vi "STED Control V8.vi"() -> ()   [LabVIEW 2014]
uses:
  Type Defs/Image Acquisition Parameters.ctl
  Laser Controls.ctl
  Detectors.ctl
  Type Defs/P541.ctl
  Type Defs/M227.ctl
  Type Defs/P612.ctl
  Type Defs/M686.ctl
  Type Defs/P841.ctl
  Type Defs/ASI.ctl
  Type Defs/N664_V2.ctl
  Type Defs/STED Graph Controls.ctl
  Type Defs/Display Controls.ctl
  FPGA-7842R-Reference.ctl
  Manual Controls V2.ctl
  Scan Parameters.ctl
  <vilib>/Utility/miscctls.llb/LVPositionTypeDef.ctl
  Controls/StageStates.ctl
  <vilib>/Utility/miscctls.llb/LVRectTypeDef.ctl
  <vilib>/event_ctls.llb/lveventtype.ctl
panel:
  out "Channel 6":sgl[][](graph)
  out "Channel 5":sgl[][](graph)
  out "Channel 4":sgl[][](graph)
  out "Channel 3":sgl[][](graph)
  out "Channel 2":sgl[][](graph)
  out "Channel 1":sgl[][](graph)
  in  "Display Controls":T1
  in  "Graph Tools":T2
  in  "Shutters":T3
  in  "Upper Objective Z - N664":T4={"Up N664"=FALSE, "Down N664"=FALSE, "Step Size (um)"=0.001, "Position (mm)"=0.0} {"Step Size (um)" min=0.001}
  in  "Load Positions":bool
  in  "Cavity Translation Z - ASI":T5={"Up ASI"=FALSE, "Down ASI"=FALSE, "Step Size (um)"=0.001, "Z (um)"=0.001, "F (um)"=0.001, "Velocity"=0.001} caption="ASI" {"Velocity" min=0.001; "F (um)" min=0.001; "Z (um)" min=-1500.0 max=1500.0; "Step Size (um)" min=0.001}
  in  "Phase Comp Mirror - P841":T6={"Position (µm)"=0.0, "Step Size (µm)"=1.0, "Up P841"=FALSE, "Down P841"=FALSE}
  in  "Sample Stage XY - M686":T7 {"Y" format="%#_4g"; "X" format="%#_4g"}
  in  "Joystick Velocity":string(combo)
  in  "Radio Buttons":enum32{"Radio Selection 1", "Radio Selection 2"}(radio)
  in  "Bottom Objective XY - P612":T8 {"Y" format="%#_4g"; "X" format="%#_4g"}
  in  "Abort AllStage":bool
  in  "Stages":T9={"M227"=TRUE, "N664"=TRUE, "P612"=TRUE, "M686"=TRUE, "P841"=TRUE, "ASI"=TRUE}
  in  "Sample Z Coarse - M227":T10
  in  "Tab Control":T11(tab)
  in  "SLM":bool
  in  "DM":bool
  in  "Timing":bool
  in  "Sample Z - P541":T12={"Step Up"=FALSE, "Step Down"=FALSE, "Z Position"=0.0, "Step Size (um)"=1.0}
  in  "Detectors":T13
  in  "Laser Controls":T14 {"STED Power (V)" scale=0.0..2.0}
  in  "Save File Path":path=path "C:/isoSTED_Data/Temp/Test_0000.dbl"
  in  "Capture":bool
  in  "Image Acquisition Parameters":T15={"Scan Type"=enum."Beam Scanning", "Scan Mode"=enum."XY", "Fast Axis Frequency (Hz)"=15780.0, "Image Format"=256, "Line Accumulations"=100, "Frames Per Capture"=1, "Frames Accumulations"=1, "Image Dimension (um)"=[15.0, 15.0], "Number of Z Steps"=1, "Z Steps Size (um)"=1.0, "Pixel Size (nm)"=[58.59375, 58.59375]} {"Z Steps Size (um)" min=0.0; "Number of Z Steps" min=1; "Frames Accumulations" min=1; "Frames Per Capture" min=1; "Line Accumulations" min=1; "Image Format" items=["64 x 64"=64, "128 x 128"=128, "256 x 256"=256, "512 x 512"=512, "1024 x 1024"=1024, "2048 x 2048"=2048]}
  in  "Live":bool
  in  "Exit":bool
  # "Sample Stage XY - M686 (0~25 mm)"
  # "XY"
  # "Z"
  # "Length"
  # "Height"
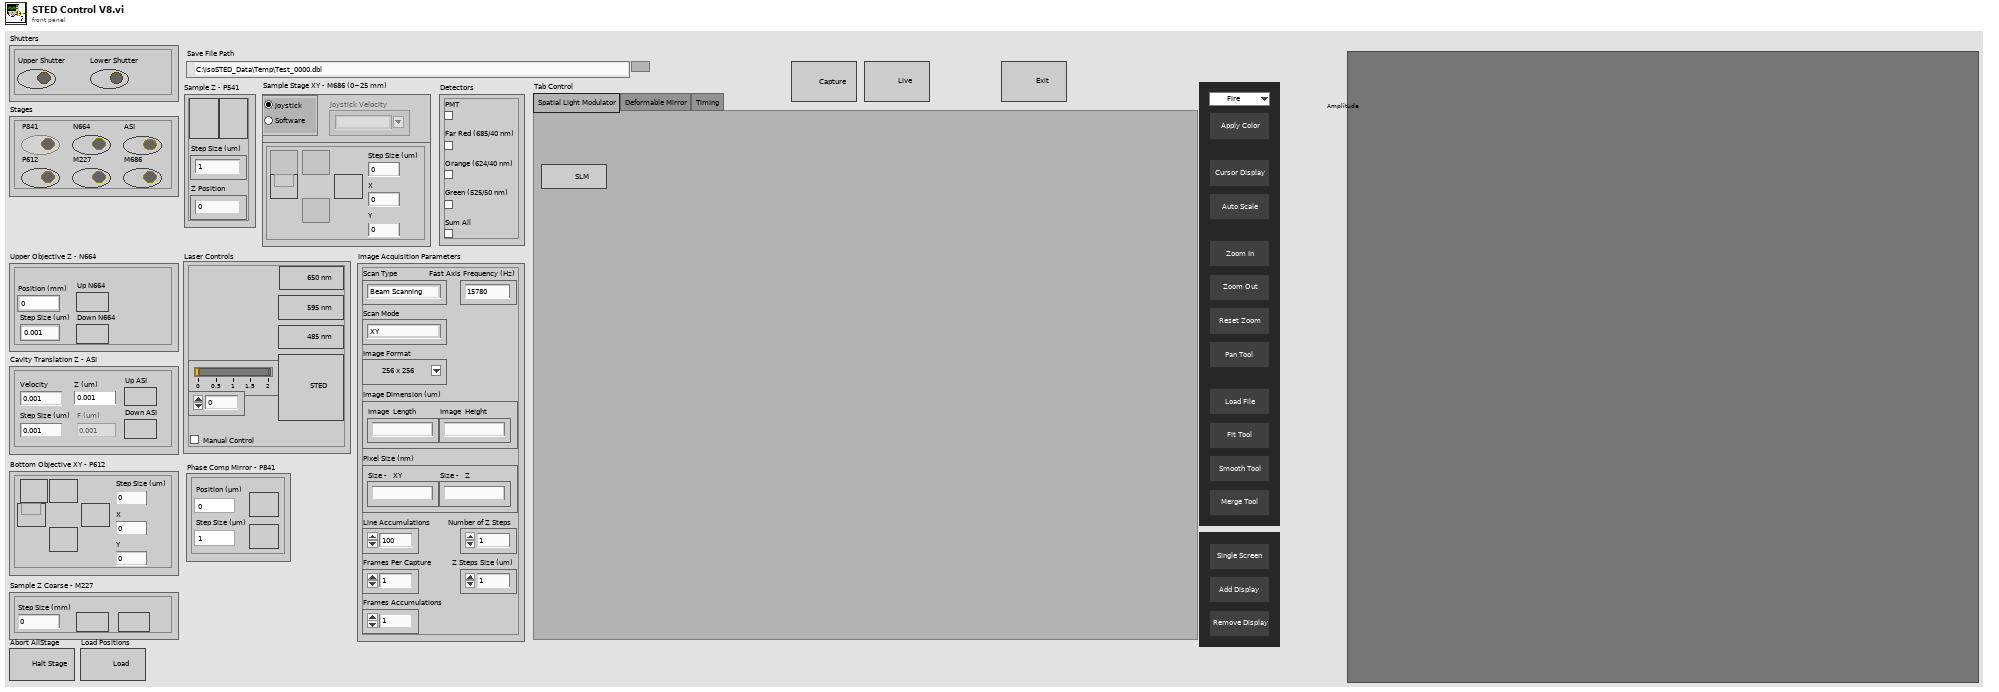
[diagram p1: front panel]
types:
  T1 = typedef "Display Controls.ctl" = cluster{"Remove Display":bool, "Add Display":bool, "Single Screen":bool}
  T2 = typedef "STED Graph Controls.ctl" = cluster{"Zoom Out":bool, "Zoom In":bool, "Reset Zoom":bool, "Pan Tool":bool, "Show Cursor":bool, "Load File":bool, "Fit Tool":bool, "Smooth Tool":bool, "Merge Tool":bool, "Auto Scale":bool, "Apply Color":bool, "Color Map":enum16{"Fire", "Gray", "Red", "Green", "Blue", "Cyan", "Magenta", "Yellow", "Red-White", "Green-White", "Blue-White", "Glow"}}
  T3 = cluster{"Upper Shutter":bool, "Lower Shutter":bool}
  T4 = typedef "N664_V2.ctl" = cluster{"Up N664":bool, "Down N664":bool, "Step Size (um)":dbl, "Position (mm)":dbl}
  T5 = typedef "ASI.ctl" = cluster{"Up ASI":bool, "Down ASI":bool, "Step Size (um)":dbl, "Z (um)":dbl, "F (um)":dbl, "Velocity":dbl}
  T6 = typedef "P841.ctl" = cluster{"Position (µm)":dbl, "Step Size (µm)":dbl, "Up P841":bool, "Down P841":bool}
  T7 = typedef "M686.ctl" = cluster{"Home Button":bool, "Up Button":bool, "Left Button":bool, "Down Button":bool, "Right Button":bool, "Step Size (um)":dbl, "X":dbl, "Y":dbl}
  T8 = typedef "P612.ctl" = cluster{"Home Button":bool, "Up Button":bool, "Left Button":bool, "Down Button":bool, "Right Button":bool, "Step Size (um)":dbl, "X":dbl, "Y":dbl}
  T9 = cluster{"M227":bool, "N664":bool, "P612":bool, "M686":bool, "P841":bool, "ASI":bool}
  T10 = typedef "M227.ctl" = cluster{"Up M227":bool, "Down M227":bool, "Step Size (mm)":dbl}
  T11 = enum32{"Spatial Light Modulator", "Deformable Mirror", "Timing"}
  T12 = typedef "P541.ctl" = cluster{"Step Up":bool, "Step Down":bool, "Z Position":dbl, "Step Size (um)":dbl}
  T13 = typedef "Detectors.ctl" = cluster{"PMT":bool, "Far Red (685/40 nm)":bool, "Orange (624/40 nm)":bool, "Green (525/50 nm)":bool, "Sum All":bool}
  T14 = typedef "Laser Controls.ctl" = cluster{"STED Power (V)":dbl, "STED":bool, "640 nm":bool, "590 nm":bool, "485 nm":bool, "Manual Control":bool}
  T15 = typedef "Image Acquisition Parameters.ctl" = cluster{"Scan Type":enum16{"Sample Scanning", "Beam Scanning"}, "Scan Mode":enum16{"XY", "XZ", "YZ", "XYZ"}, "Fast Axis Frequency (Hz)":dbl, "Image Format":u16, "Line Accumulations":u16, "Frames Per Capture":u16, "Frames Accumulations":u16, "Image Dimension (um)":dbl[], "Number of Z Steps":u8, "Z Steps Size (um)":dbl, "Pixel Size (nm)":dbl[]}
  T16 = typedef "Scan Parameters.ctl" = cluster{"Fast_Ax_Amp_V":dbl, "Fast_Ax_Off_V":dbl, "Slow_Ax_Amp_V":dbl, "Slow_Ax_Off_V ":dbl, "Slow_Ax_Max_V_VperS":dbl, "Slow_Ax1_Del25ns":i32, "Slow_Ax2_Del25ns":i32, "Stage_X_Off_V":dbl, "Stage_Y_Off_V":dbl, "Stage_Z_Off_V":dbl, "Galvo1_Off_V":dbl, "Galvo2_Off_V":dbl, "Last_Scan_Mode":enum16{"XY", "XZ", "YZ", "XYZ"}, "Current_Scan_Mode":enum16{"XY", "XZ", "YZ", "XYZ"}, "Fly_Back_Lines":u16, "Linear_Ramp_End":u32, "Z_Step_I16":i16, "Z_Start_I16":i16, "Laser_States _U32":u32, "590_Voltage_I16":i16, "775_AOM_Volt_I16":i16, "Blanking OFF":bool, "Unused_Axis_I16":i16}
  T17 = typedef "Manual Controls V2.ctl" = cluster{"Galvo 1 Position (I16)":i16, "Galvo 2 Position (I16)":i16, "X Axis Voltage (I16)":i16, "Y Axis Voltage (I16)":i16, "Z Axis Voltage (I16)":i16, "Res Mirror Amp (I16)":i16, "Res Mirror Mute":bool, "Upper Shutter":bool, "Lower Shutter":bool}
  T18 = typedef "FPGA-7842R-Reference.ctl" = enum16{"Stage Control", "Laser Control", "Unused Axis I16", "Exit", "Set Res Mirror", "Set Galvo", "Default", "Close FPGA", "Stop Waveforms", "Start Waveforms", "Shutter Control", "Initialize"}
  T19 = enum8{"Enabled", "Disabled", "Disabled and Grayed Out"}
  T20 = typedef "StageStates.ctl" = enum16{"POSITION", "MVR", "MOVE", "HALT", "ONTARGET", "ERROR", "EXIT", "HOME", "ZEROPOS", "NANOPOS", "QUIT", "ANALOG"}
  T21 = typedef "LVRectTypeDef.ctl" = cluster{"Left":i16, "Top":i16, "Right":i16, "Bottom":i16}
  T22 = enum32{"Invalid", "Standard", "Closed", "Hidden", "Minimized", "Maximized"}
  T23 = typedef "lveventtype.ctl" = enum32{"Null", "Timeout", "Annotation Menu Selection", "Annotation Menu Selection?", "App Instance Close", "App Instance Close?", "Autoscale Range Change", "Bookmark Info Change", "Cell Edit", "Cell Edit?", "Cursor Grab", "Cursor Grab?", "Cursor Menu Selection", "Cursor Menu Selection?", "Cursor Move", "Cursor Release", "Data Change", "Direction Change", "Display State Change", "Drag Ended", "Drag Enter", "Drag Leave", "Drag Over", "Drag Source Update", "Drag Starting", "Drag Starting?", "Drop", "Exec State Change", "Key Down", "Key Down?", "Key Repeat", "Key Repeat?", "Key Up", "Listbox Double Click", "Menu Activation?", "Menu Selection (App)", "Menu Selection? (App)", "Menu Selection (User)", "Mouse Down", "Mouse Down?", "Mouse Enter", "Mouse Leave", "Mouse Move", "Mouse Up", "Mouse Wheel", "NI Security User Change (App)", "Pane Size", "Panel Close", "Panel Close?", "Panel Resize", "Plot Attribute Change", "Scale Range Change", "Shortcut Menu Activation?", "Shortcut Menu Selection (App)", "Shortcut Menu Selection? (App)", "Shortcut Menu Selection (User)", "Tree Double Click", "Tree Drag", "Tree Drag?", "Tree Drop", "Tree Drop?", "Tree Item Close", "Tree Item Close?", "Tree Item Open", "Tree Item Open?", "User Event", "Value Change"}
  T24 = typedef "LVPositionTypeDef.ctl" = cluster{"Left":i32, "Top":i32}
  T25 = enum16{"open", "open or create", "create or replace", "create", "open (read-only)"}
  T26 = cluster{"Upper Shutter":bool, "Upper Shutter":bool}
  T27 = cluster{"Down_N664":bool, "Down_N664":bool, "Step Size (um)":dbl, "Numeric":dbl}
  T28 = cluster{bool, bool, bool, bool, bool, dbl, "Numeric":dbl, "Numeric":dbl}
  T29 = cluster{"Scan Type":bool, "Scan Mode":bool, "Fast Axis Frequency (Hz)":bool, "Image Format":bool, "Line Accumulations":bool, "Frames Per Capture":bool, "Frames Accumulations":bool, "Image Dimension (um)":bool[], "Number of Z Steps":bool, "Z Steps Size (um)":bool, "Pixel Size (nm)":bool[]}
  T30 = typedef "LVAllMonitorsDisplayTypeDef.ctl" = cluster{"Bounds":cluster{"Left":i16, "Top":i16, "Right":i16, "Bottom":i16}, "Depth":i16}[]
  T31 = cluster{"Bounds":cluster{"Left":i16, "Top":i16, "Right":i16, "Bottom":i16}, "Depth":i16}
  T32 = enum16{"Fire", "Gray", "Red", "Green", "Blue", "Cyan", "Magenta", "Yellow", "Red-White", "Green-White", "Blue-White", "Glow"}
  T33 = typedef "LVPointDoubleTypeDef.ctl" = cluster{"Cursor X":dbl, "Cursor Y":dbl}
  T34 = typedef "LVRangeTypeDef.ctl" = cluster{"Minimum":dbl, "Maximum":dbl, "Increment":dbl, "Minor Increment":dbl, "Start":dbl}
  T35 = typedef "IMAQ Image.ctl" = refnum<image>
  T36 = typedef "Waveform Data.ctl" = cluster{"Waveform Scan Parameters":cluster{"Scanning Mode":u8, "Fast Axis WF Length (Elements)":i32, "Fast Axis Sample Period (Ticks)":u32, "Slow Axis 1 WF Length (Elements)":i32, "Slow Axis 1 Sample Period (Ticks)":u32, "Slow Axis 1 Delay (25 ns) Steps":i32, "Slow Axis 2 WFLength (Elements)":i32, "Slow Axis 2 Sample Period (Ticks)":u32, "Slow Axis 2 Delay (25 ns) Steps":i32}, "Fast Axis Waveform":dbl[], "Slow Axis 1 Waveform":dbl[], "Slow Axis 2 Waveform":dbl[]}
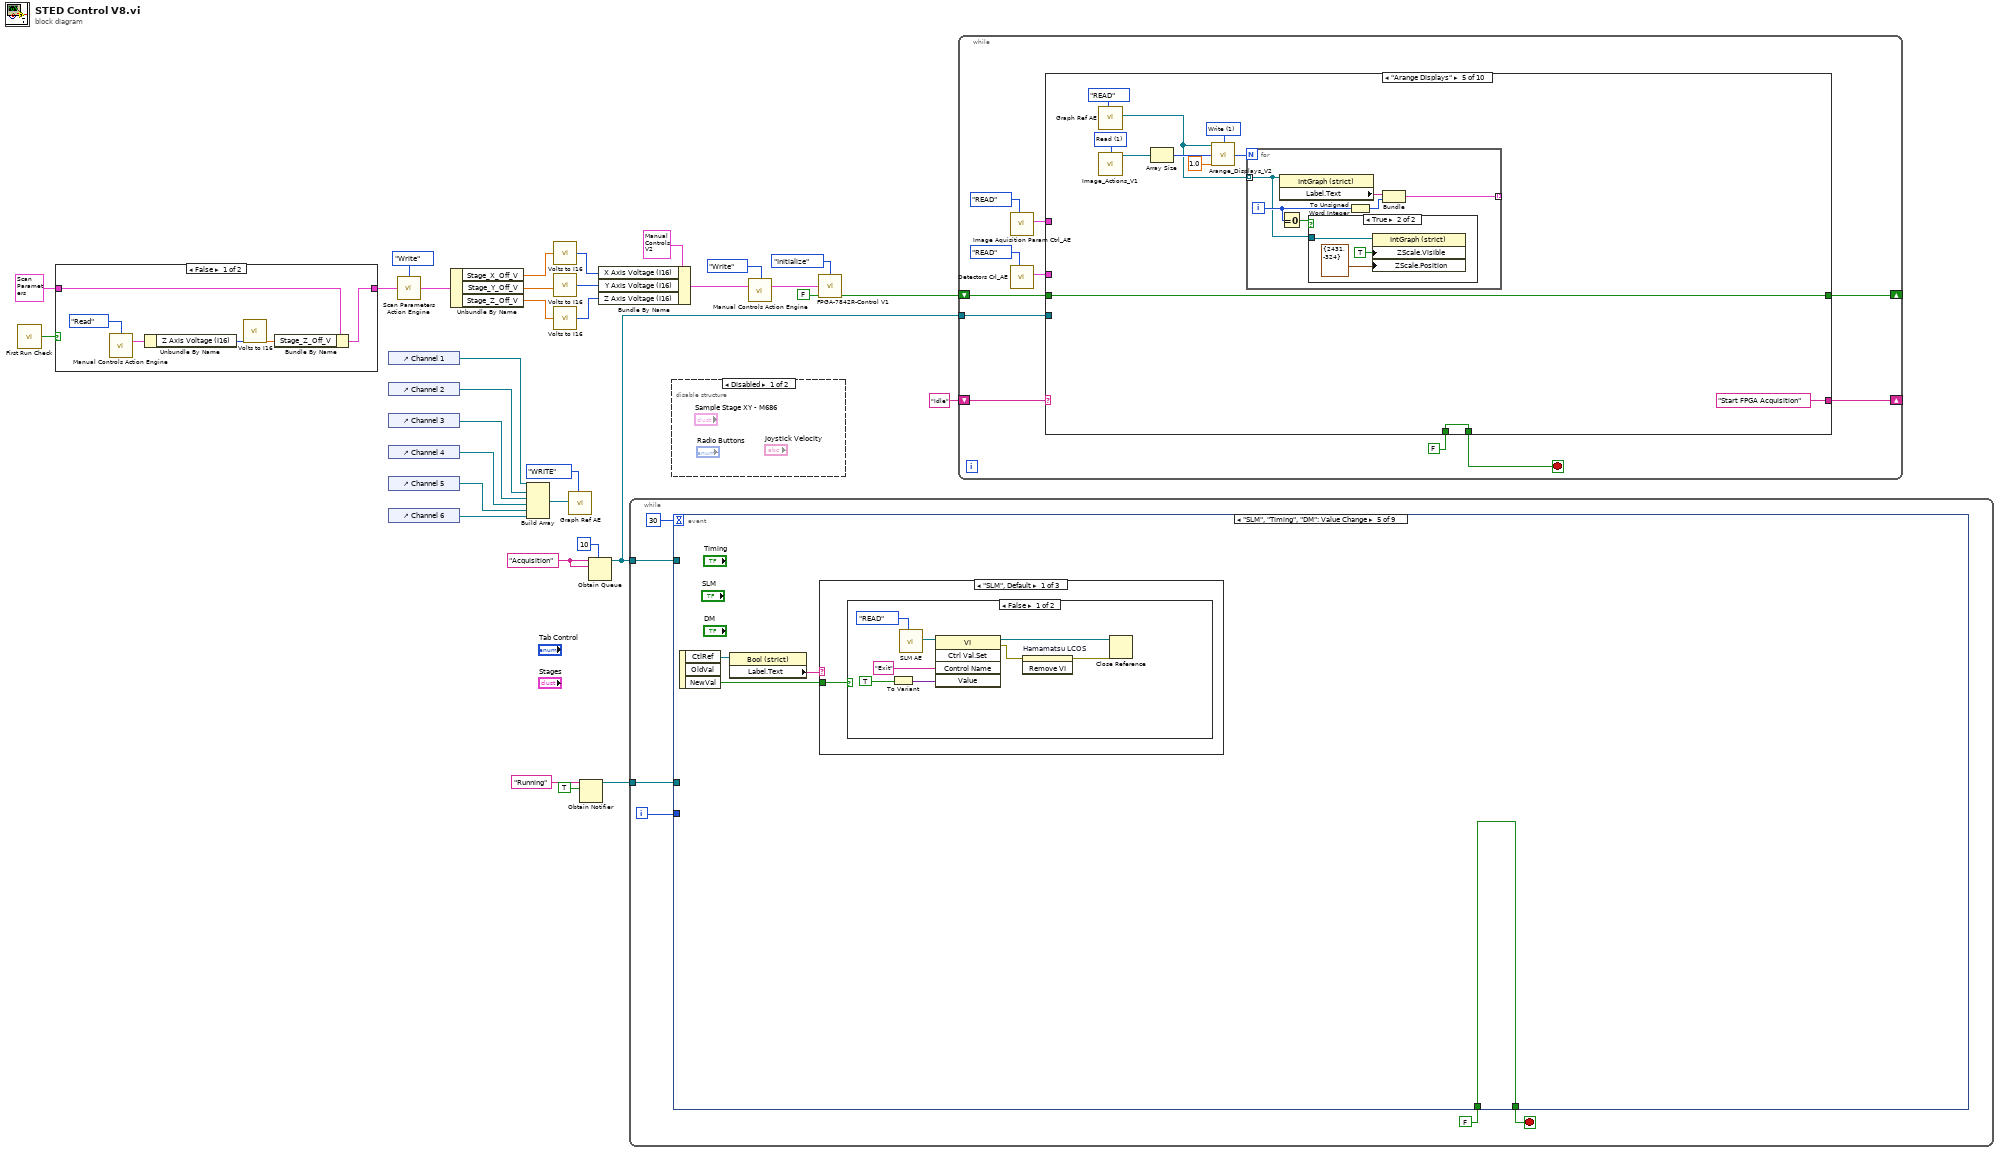
[diagram p0: block diagram]
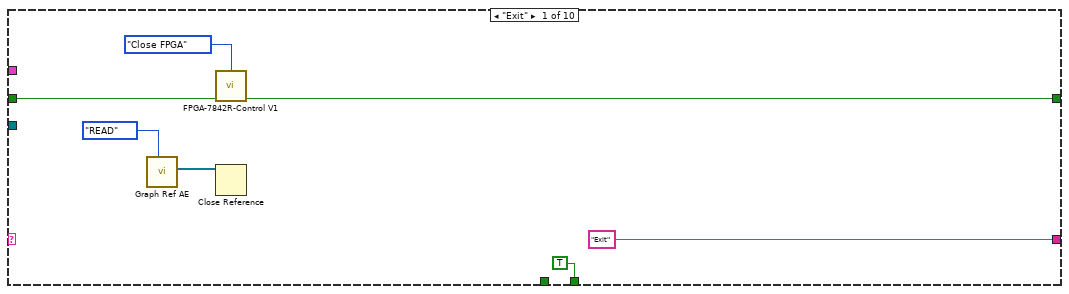
[diagram p4: hidden frame]
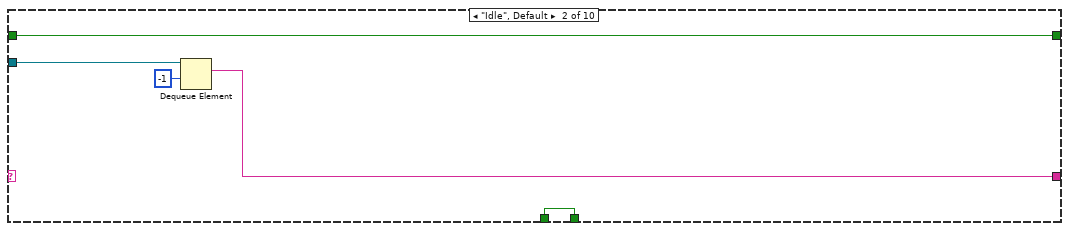
[diagram p5: hidden frame]
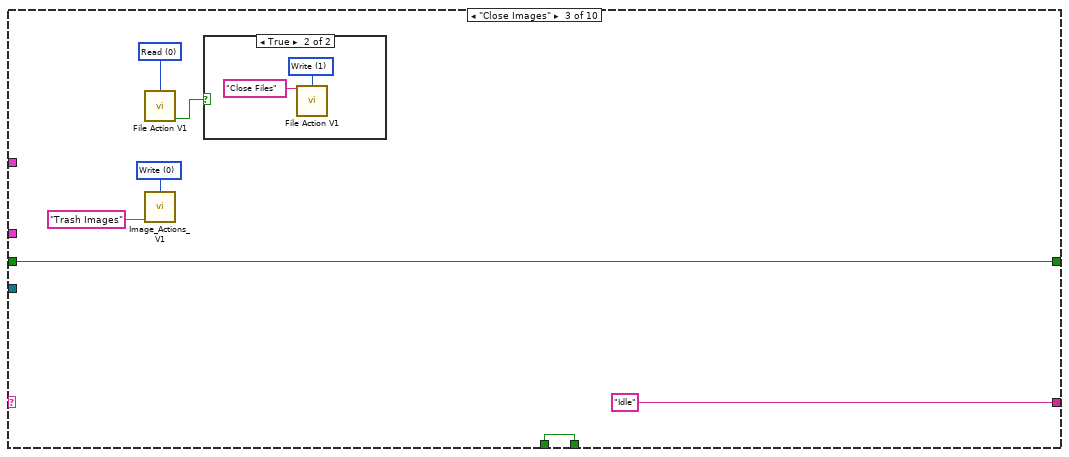
[diagram p6: hidden frame]
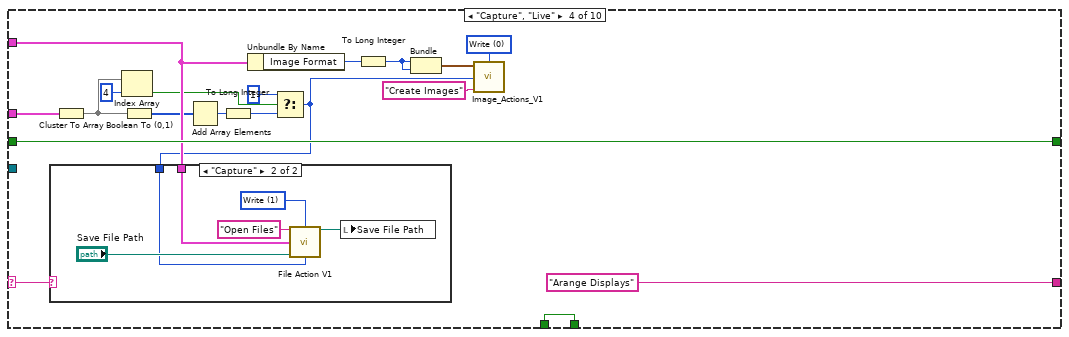
[diagram p8: hidden frame]
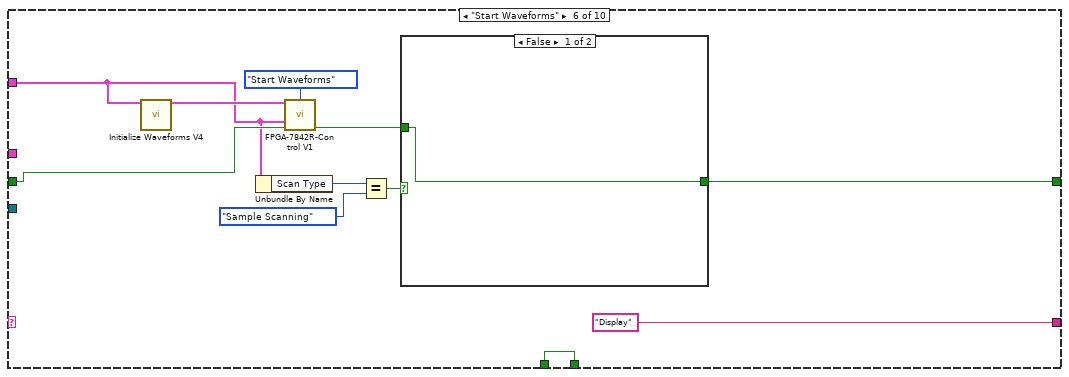
[diagram p11: hidden frame]
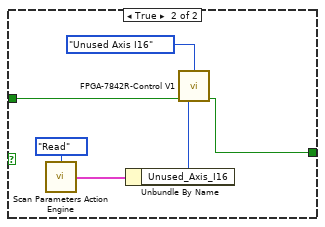
[diagram p12: hidden frame]
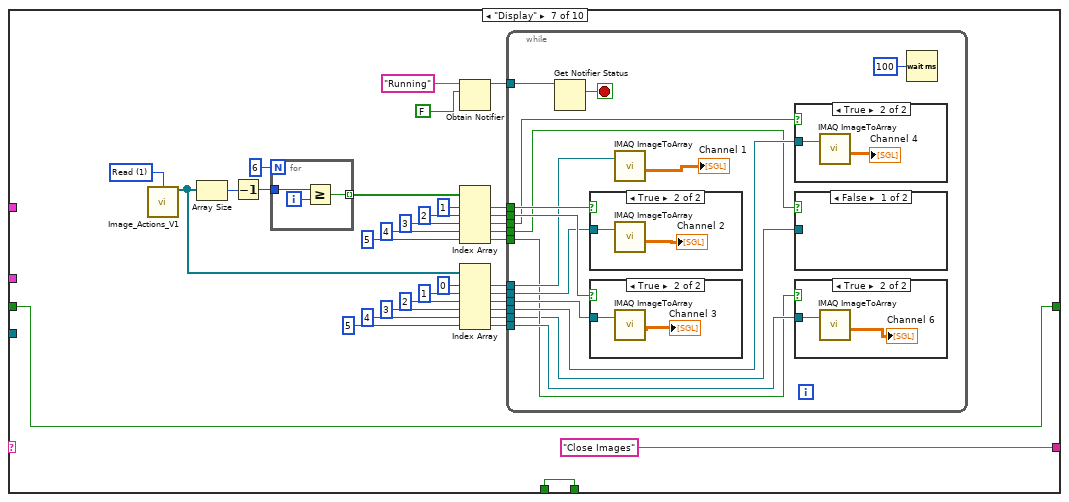
[diagram p13: hidden frame]
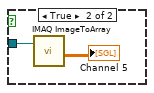
[diagram p15: hidden frame]
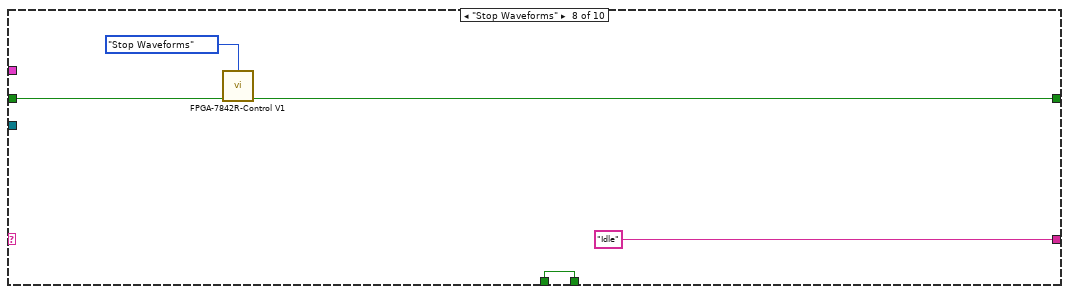
[diagram p19: hidden frame]
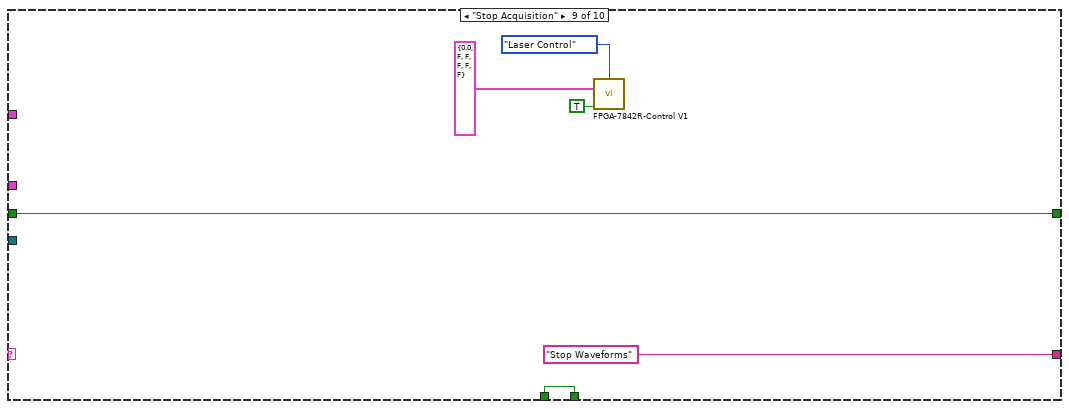
[diagram p20: hidden frame]
diagram:
  w16 = "Acquisition" ("name (unnamed)")
  n1 = call "First Run Check.vi"() -> ("First Run?"=w10:bool)  [unwired: 15 in]
  n2 = case shown="False" w10 {
    tunnel: T16 {"Fast_Ax_Amp_V"=0.0, "Fast_Ax_Off_V"=0.0, "Slow_Ax_Amp_V"=0.0, "Slow_Ax_Off_V "=0.0, "Slow_Ax_Max_V_VperS"=0.0, "Slow_Ax1_Del25ns"=0, "Slow_Ax2_Del25ns"=0, "Stage_X_Off_V"=5.0, "Stage_Y_Off_V"=5.0, "Stage_Z_Off_V"=5.0, "Galvo1_Off_V"=0.0, "Galvo2_Off_V"=0.0, "Last_Scan_Mode"=enum."XY", "Current_Scan_Mode"=enum."XY", "Fly_Back_Lines"=0, "Linear_Ramp_End"=0, "Z_Step_I16"=0, "Z_Start_I16"=0, "Laser_States _U32"=0, "590_Voltage_I16"=0, "775_AOM_Volt_I16"=0, "Blanking OFF"=FALSE, "Unused_Axis_I16"=16384} ("Scan Parameters IN") -> [w39 w40]
    tunnel: [w34 w40] -> w8
    frame False {
      n3 = call "Manual Controls Action Engine.vi"("Action"=enum16{"Read", "Write"}."Read") -> ("Manual Controls Out"=w37:T17)  [unwired: 14 in]
      n4 = Unbundle By Name(w37) -> ("Z Axis Voltage (I16)"=w38:i16)
      n5 = call "Volts to I16.vi"("Volatge (I16)"=w38) -> ("Voltage (V)"=w35:dbl)  [unwired: 13 in, 1 out]
      n6 = Bundle By Name(cluster=w39, "Stage_Z_Off_V"=w35) -> (w34:T16)
    }
    frame True {
    }
  }
  n7 = control-ref of="Channel 1"() -> (w5:refnum<vi>)
  n8 = control-ref of="Channel 2"() -> (w6:refnum<vi>)
  n9 = control-ref of="Channel 3"() -> (w7:refnum<vi>)
  n10 = control-ref of="Channel 4"() -> (w2:refnum<vi>)
  n11 = control-ref of="Channel 5"() -> (w4:refnum<vi>)
  n12 = control-ref of="Channel 6"() -> (w3:refnum<vi>)
  n13 = call "Scan Parameters Action Engine.vi"("Action"=enum16{"Read", "Write"}."Write", "Scan Parameters IN"=w8) -> ("Scan Parameters OUT"=w26:T16)  [unwired: 13 in]
  n14 = Unbundle By Name(w26) -> ("Stage_X_Off_V"=w22:dbl, "Stage_Y_Off_V"=w21:dbl, "Stage_Z_Off_V"=w20:dbl)
  n15 = Build Array(w5, w6, w7, w2, w4, w3) -> (w1:refnum<vi>[])
  n16 = call "Volts to I16.vi"("Voltage (V)"=w22) -> ("I16"=w23:i16)  [unwired: 13 in, 1 out]
  n17 = call "Volts to I16.vi"("Voltage (V)"=w21) -> ("I16"=w24:i16)  [unwired: 13 in, 1 out]
  n18 = call "Volts to I16.vi"("Voltage (V)"=w20) -> ("I16"=w25:i16)  [unwired: 13 in, 1 out]
  n19 = call "Graph Ref AE.vi"("Action"=enum16{"READ", "WRITE"}."WRITE", "Graph Ref In"=w1) -> ()  [unwired: 9 in, 1 out]
  n20 = Obtain Notifier(name (unnamed)="Running", notification data type=TRUE) -> (notifier out=w12:refnum<notifier>)  [unwired: 2 in, 2 out]
  n21 = Obtain Queue(max queue size (-1, unlimited)=10, name (unnamed)=w16, element data type=w16) -> (queue out=w18:refnum<queue>)  [unwired: 2 in, 2 out]
  n22 = Bundle By Name(cluster=T17 {"Galvo 1 Position (I16)"=-280, "Galvo 2 Position (I16)"=0, "X Axis Voltage (I16)"=16384, "Y Axis Voltage (I16)"=16384, "Z Axis Voltage (I16)"=16384, "Res Mirror Amp (I16)"=0, "Res Mirror Mute"=FALSE, "Upper Shutter"=FALSE, "Lower Shutter"=FALSE} ("Manual Controls"), "X Axis Voltage (I16)"=w23, "Y Axis Voltage (I16)"=w24, "Z Axis Voltage (I16)"=w25) -> (w27:T17)
  n23 = while {
    tunnel: w18 -> [w44]
    tunnel: w12 -> [w41]
    i -> [w42]
    stop <- w46 stop-if-true
    n24 = event shown="[4] \"SLM\", \"Timing\", \"DM\": Value Change" {
      selector: _ -> [_ _ _ _ _ _ _ _ _]
      dyn-events: _ -> [_ _ _ _ _ _ _ _ _]
      timeout: 30 -> [_ _ _ _ _ _ _ _ _]
      tunnel: [w54 w154 w167 w293 w522 w573 w767 w803 w904] -> w46
      tunnel: FALSE -> [w54 w154 w167 w293 w522 w573 w767 w803 _]
      tunnel: w44 -> [w51 w153 _ _ _ _ _ _ w903]
      tunnel: w42 -> [w49 _ _ _ _ _ _ _ _]
      tunnel: w41 -> [w47 w146 _ _ _ _ _ _ w897]
      event Timeout {
        n25 = event-data() -> ()  [unwired: 1 in, 3 out]
        n26 = Equal To 0?(x=w49) -> (x = 0?=w48:bool)
        n27 = Get Notifier Status(notifier=w47) -> (current notification=w53:bool)  [unwired: 1 in, 4 out]
        n28 = case shown="False" w48 {
          frame False {
            w59 = enum16{"WRITE", "READ"}."READ" ("Enum")
            n29 = call "Image Aquisition Param Ctrl_AE.vi"("Action"=enum16{"READ", "WRITE"}."READ") -> ("Image Acquisition Parameters Out"=w75:T15)  [unwired: 10 in]
            n30 = call "Detectors Crl_AE.vi"("Action"=enum16{"READ", "WRITE"}."READ") -> ("Detectors Parameters Out"=w76:T13)  [unwired: 10 in]
            n31 = call "LASERs_ Crl_AE.vi"("Action"=enum16{"READ", "WRITE"}."READ") -> ("Detectors Parameters Out"=w77:T14)  [unwired: 10 in]
            n32 = local write "Image Acquisition Parameters"(w75) -> ()
            n33 = local write "Detectors"(w76) -> ()
            n34 = local write "Laser Controls"(w77) -> ()
            n35 = call "Stage_position_ae.vi"("StageID"="P612", "Enum"=w59) -> ("Position Out"=w70:dbl[])  [unwired: 8 in, 1 out]
            n36 = call "Stage_position_ae.vi"("StageID"="P841", "Enum"=w59) -> ("Position Out"=w63:dbl[])  [unwired: 8 in, 1 out]
            n37 = call "Stage_position_ae.vi"("StageID"="N664", "Enum"=w59) -> ("Position Out"=w56:dbl[])  [unwired: 8 in, 1 out]
            n38 = Index Array(array=w56, index=0) -> (element=w55:dbl)
            n39 = Index Array(array=w63, index=0) -> (element=w60:dbl)
            n40 = Index Array(array=w70, index #1=0 ("index"), index #2=1 ("index"), index #3=2 ("index")) -> (element #1=w69:dbl, element #2=w66:dbl, element #3=w64:dbl)
            n41 = property on="Position (µm)" class="DigNum (strict)"("Value"=w60) -> ()  [unwired: 2 in, 2 out]
            n42 = property on="Position (mm)" class="DigNum (strict)"("Value"=w55) -> ()  [unwired: 2 in, 2 out]
            n43 = property on="X" class="DigNum (strict)"("Value"=w69) -> ()  [unwired: 2 in, 2 out]
            n44 = property on="Y" class="DigNum (strict)"("Value"=w66) -> ()  [unwired: 2 in, 2 out]
            n45 = property on="Z Position" class="DigNum (strict)"("Value"=w64) -> ()  [unwired: 2 in, 2 out]
          }
          frame True {
            w78 = FALSE ("Upper Shutter")
            n46 = local read "Image Acquisition Parameters"() -> (w85:T15)
            n47 = local read "Laser Controls"() -> (w83:T14)
            n48 = local read "Detectors"() -> (w82:T13)
            n49 = Bundle("Upper Shutter"=w78, "Upper Shutter"=w78) -> (w79:T26)  [unwired: 1 in]
            n50 = property on="Shutters" class="Clust (strict)"("Value"=w79) -> ()  [unwired: 2 in, 2 out]
            n51 = call "Image Aquisition Param Ctrl_AE.vi"("Action"=enum16{"READ", "WRITE"}."WRITE", "Image Acquisition Parameters In"=w85) -> ()  [unwired: 9 in, 1 out]
            n52 = call "Detectors Crl_AE.vi"("Action"=enum16{"READ", "WRITE"}."WRITE", "Detectors Parameters In"=w82) -> ()  [unwired: 9 in, 1 out]
            n53 = call "LASERs_ Crl_AE.vi"("Action"=enum16{"READ", "WRITE"}."WRITE", "Detectors Parameters In"=w83) -> ()  [unwired: 9 in, 1 out]
            n54 = property on="Stages" class="Clust (strict)"() -> ("Controls[]"=w80:refnum<vi>[])  [unwired: 2 in, 2 out]
            n55 = for {
              tunnel: w80 -> [w90] mode=indexing
              n56 = property class="Ctl"(reference=w90) -> ("Label.Text"=w88:string, "Value"=w92:variant)  [unwired: 1 in, 2 out]
              n57 = Variant To Data(type=TRUE, Variant=w92) -> (data=w89:bool)  [unwired: 1 in, 1 out]
              n58 = call "All_Stages_Aloha.vi"("Aloha"=w89, "Stage ID"=w88) -> ("Position Out"=w87:dbl[])  [unwired: 9 in]
              n59 = case shown="\"P612\"" w88 {
                tunnel: w87 -> [_ _ w99 w106 w116 w127 w137]
                frame "0", Default {
                }
                frame "M227" {
                  w96 = FALSE
                  n60 = Bundle(w96, w96, 0.0) -> (w94:cluster{bool, bool, dbl})  [unwired: 1 in]
                  n61 = To Variant(anything=w94) -> (Variant=w93:variant)
                  n62 = property on="Sample Z Coarse - M227" class="Clust"("Value"=w93) -> ()  [unwired: 2 in, 2 out]
                }
                frame "N664" {
                  w102 = FALSE ("Down_N664")
                  n63 = Index Array(array=w99, index=0) -> (element=w100:dbl)
                  n64 = Bundle("Down_N664"=w102, "Down_N664"=w102, "Step Size (um)"=1.0, "Numeric"=w100) -> (w98:T27)  [unwired: 1 in]
                  n65 = To Variant(anything=w98) -> (Variant=w97:variant)
                  n66 = property on="Upper Objective Z - N664" class="Clust"("Value"=w97) -> ()  [unwired: 2 in, 2 out]
                }
                frame "P612" {
                  w114 = FALSE
                  n67 = Index Array(array=w106, index #1=0, index #2=1, index #3=2 ("index")) -> (element #1=w111:dbl, element #2=w109:dbl, element #3=w104:dbl)
                  n68 = Bundle(w114, w114, w114, w114, w114, 1.0, "Numeric"=w111, "Numeric"=w109) -> (w110:T28)  [unwired: 1 in]
                  n69 = To Variant(anything=w110) -> (Variant=w105:variant)
                  n70 = property on="Bottom Objective XY - P612" class="Clust"("Value"=w105) -> ()  [unwired: 2 in, 2 out]
                  n71 = property on="Z Position" class="DigNum (strict)"("Value"=w104) -> ()  [unwired: 2 in, 2 out]
                }
                frame "M686" {
                  w125 = FALSE
                  n72 = Index Array(array=w116, index #1=0, index #2=1) -> (element #1=w122:dbl, element #2=w117:dbl)
                  n73 = Bundle(w125, w125, w125, w125, w125, 10.0, "Numeric"=w122, "Numeric"=w117) -> (w121:T28)  [unwired: 1 in]
                  n74 = To Variant(anything=w121) -> (Variant=w115:variant)
                  n75 = property on="Joystick Velocity" class="CmbBox"("DisabledEnum"=T19."Disabled and Grayed Out" ("Disabled")) -> ()  [unwired: 2 in, 2 out]
                  n76 = property on="Radio Buttons" class="RadioBtnsControl (strict)"("Value"=enum32{"Radio Selection 1", "Radio Selection 2"}."Radio Selection 2" ("Radio Buttons")) -> ()  [unwired: 2 in, 2 out]
                  n77 = property on="Sample Stage XY - M686" class="Clust"("Value"=w115) -> ()  [unwired: 2 in, 2 out]
                }
                frame "P841" {
                  n78 = Index Array(array=w127, index=0) -> (element=w126:dbl)
                  n79 = property on="Position (µm)" class="DigNum (strict)"("Value"=w126) -> ()  [unwired: 2 in, 2 out]
                }
                frame "ASI" {
                  w133 = FALSE
                  n80 = Add Array Elements(numeric array=w137) -> (sum=w139:dbl)
                  n81 = Index Array(array=w137, index #1=0 ("index"), index #2=1 ("index")) -> (element #1=w132:dbl, element #2=w131:dbl)
                  n82 = Divide(x=w139, y=2000.0) -> ()  [unwired: 1 out]
                  n83 = Bundle By Name(cluster=T5 {"Up ASI"=FALSE, "Down ASI"=FALSE, "Step Size (um)"=0.001, "Z (um)"=0.001, "F (um)"=0.001, "Velocity"=0.001} ("Cavity Translation Z - ASI"), "Up ASI"=w133, "Down ASI"=w133, "Step Size (um)"=1.0, "Z (um)"=w132, "F (um)"=w131, "Velocity"=0.1) -> (w129:T5)
                  n84 = To Variant(anything=w129) -> (Variant=w130:variant)
                  n85 = property on="Cavity Translation Z - ASI" class="Clust"("Value"=w130) -> ()  [unwired: 2 in, 2 out]
                }
              }
            }
          }
        }
        n86 = local read "Capture"() -> (w52:bool)
        n87 = And(x=w53, y=w52) -> (x .and. y?=w50:bool)
        n88 = case shown="False" w50 {
          tunnel: w51 -> [_ w144]
          frame False {
          }
          frame True {
            n89 = local write "Capture"(FALSE ("Capture")) -> ()
            n90 = Enqueue Element(queue=w144, element="Stop Acquisition" ("f")) -> ()  [unwired: 2 in, 3 out]
            n91 = property on="Live" class="Bool (strict)"("DisabledEnum"=T19."Enabled" ("Disabled")) -> ()  [unwired: 2 in, 2 out]
          }
        }
      }
      event "Live", "Capture": Value Change {
        n92 = event-data() -> ("CtlRef"=w152:refnum<vi>, "NewVal"=w147:bool)  [unwired: 1 in]
        n93 = Not(x=w147) -> (.not. x?=w150:bool)
        n94 = property class="Bool (strict)"(reference=w152) -> ("Label.Text"=w148:string)  [unwired: 1 in, 2 out]
        n95 = Send Notification(notification=w150, notifier=w146) -> ()  [unwired: 1 in, 2 out]
        n96 = case shown="\"Live\"" w148 {
          tunnel: w147 -> [_ w156 w160]
          frame "False", Default {
          }
          frame "Live" {
            n97 = case shown="True" w156 {
              tunnel: [T19."Enabled" ("Disabled") T19."Disabled and Grayed Out" ("Disabled")] -> w155
              frame False {
              }
              frame True {
              }
            }
            n98 = property on="Capture" class="Bool (strict)"("DisabledEnum"=w155) -> ()  [unwired: 2 in, 2 out]
            n99 = property on="Exit" class="Bool"("DisabledEnum"=w155) -> ()  [unwired: 2 in, 2 out]
          }
          frame "Capture" {
            n100 = case shown="True" w160 {
              tunnel: [T19."Enabled" ("Disabled") T19."Disabled and Grayed Out" ("Disabled")] -> w159
              frame False {
              }
              frame True {
              }
            }
            n101 = property on="Live" class="Bool (strict)"("DisabledEnum"=w159) -> ()  [unwired: 2 in, 2 out]
            n102 = property on="Exit" class="Bool"("DisabledEnum"=w159) -> ()  [unwired: 2 in, 2 out]
          }
        }
        n103 = Select(t=w148, s=w147, f="Stop Acquisition") -> (s? t:f=w149:string)
        n104 = Enqueue Element(queue=w153, element=w149) -> ()  [unwired: 2 in, 3 out]
      }
      event "Shutters": Value Change {
        n105 = event-data() -> ("CtlRef"=w166:refnum<vi>, "NewVal"=w165:variant, "OldVal"=w164:variant)  [unwired: 1 in]
        n106 = property class="Clust"(reference=w166) -> ("Label.Text"=w163:string)  [unwired: 1 in, 2 out]
        n107 = case shown="\"Shutters\"" w163 {
          tunnel: w165 -> [_ w178 _ _ _]
          tunnel: w164 -> [_ w176 _ _ _]
          frame Default {
          }
          frame "Image Acquisition Parameters" {
            n108 = Variant To Data(type="Image Acquisition Parameters", Variant=w178) -> (data=w175:T15)  [unwired: 1 in, 1 out]
            n109 = Variant To Data(type=w175, Variant=w176) -> (data=w174:T15)  [unwired: 1 in, 1 out]
            n110 = Not Equal?(x=w175, y=w174) -> (x != y?=w200:T29)
            n111 = Unbundle By Name(w200) -> ("Image Dimension (um)"=w185:bool[], "Image Format"=w183:bool, "Pixel Size (nm)"=w184:bool[])
            n112 = Or Array Elements(Boolean array=w185) -> (logical OR=w189:bool)
            n113 = Or Array Elements(Boolean array=w184) -> (logical OR=w188:bool)
            n114 = Build Array(w189, w183, w188) -> (w187:bool[])
            n115 = Boolean Array To Number(Boolean array=w187) -> (number=w186:u32)
            n116 = case shown="1, 2" w186 {
              tunnel: w185 -> [_ w222 _]
              tunnel: w175 -> [w210 w215 w230]
              tunnel: [w210 w213 w228] -> w182
              tunnel: w184 -> [_ _ w227]
              tunnel: [w209 w212 w226] -> w181
              tunnel: [w208 w211 w225] -> w179
              frame 0, Default {
                n117 = Unbundle By Name(w210) -> ("Image Dimension (um)"=w209:dbl[], "Scan Mode"=w208:enum16{"XY", "XZ", "YZ", "XYZ"})
              }
              frame 1, 2 {
                # "Image Dimension or Format Change"
                n118 = Unbundle By Name(w215) -> ("Image Dimension (um)"=w221:dbl[], "Image Format"=w219:u16, "Scan Mode"=w211:enum16{"XY", "XZ", "YZ", "XYZ"})
                n119 = for {
                  tunnel: w222 -> [w224] mode=indexing
                  tunnel: w221 -> [w223] mode=indexing
                  tunnel: [w223] -> w220
                  stop <- w224 stop-if-true
                }
                n120 = To Double Precision Float(number=w219) -> (double precision float=w218:dbl)
                n121 = Build Array(w220, w220) -> (w212:dbl[])
                n122 = Divide(x=w212, y=w218) -> (x/y=w217:dbl[])
                n123 = Multiply(x=w217, y=1000.0) -> (x*y=w214:dbl[])
                n124 = Bundle By Name(cluster=w215, "Image Dimension (um)"=w212, "Pixel Size (nm)"=w214) -> (w213:T15)
              }
              frame 4 {
                # "Pixel Size Change"
                n125 = Unbundle By Name(w230) -> ("Pixel Size (nm)"=w236:dbl[], "Image Format"=w234:u16, "Scan Mode"=w225:enum16{"XY", "XZ", "YZ", "XYZ"})
                n126 = for {
                  tunnel: w227 -> [w238] mode=indexing
                  tunnel: w236 -> [w237] mode=indexing
                  tunnel: [w237] -> w235
                  stop <- w238 stop-if-true
                }
                n127 = Build Array(w235, w235) -> (w229:dbl[])
                n128 = To Double Precision Float(number=w234) -> (double precision float=w233:dbl)
                n129 = Multiply(x=w229, y=w233) -> (x*y=w232:dbl[])
                n130 = Multiply(x=w232, y=0.001) -> (x*y=w226:dbl[])
                n131 = Bundle By Name(cluster=w230, "Pixel Size (nm)"=w229, "Image Dimension (um)"=w226) -> (w228:T15)
              }
            }
            n132 = Index Array(array=w181, index=0) -> (element=w205:dbl)
            n133 = Not Equal?(x=enum16{"XY", "XZ", "YZ", "XYZ"}."YZ" ("y"), y=w179) -> (x != y?=w190:bool)
            n134 = call "Res Mirror um to Volts.vi"("Image Size (um)"=w205) -> ("Voltage (V)"=w168:dbl)
            n135 = Select(t=15780.0, s=w190, f=200.0) -> (s? t:f=w193:dbl)
            n136 = In Range and Coerce(upper limit=5.0, x=w168, lower limit=0.0) -> (coerced(x)=w170:dbl)  [unwired: 1 out]
            n137 = call "Scan Parameters Action Engine.vi"("Action"=enum16{"Read", "Write"}."Read") -> ("Scan Parameters OUT"=w171:T16)  [unwired: 14 in]
            n138 = Bundle By Name(cluster=w171, "Fast_Ax_Amp_V"=w170) -> (w169:T16)
            n139 = Bundle By Name(cluster=w182, "Fast Axis Frequency (Hz)"=w193) -> (w192:T15)
            n140 = call "Volts to I16.vi"("Voltage (V)"=w170) -> ("I16"=w204:i16)  [unwired: 13 in, 1 out]
            n141 = call "Scan Parameters Action Engine.vi"("Action"=enum16{"Read", "Write"}."Write", "Scan Parameters IN"=w169) -> ()  [unwired: 13 in, 1 out]
            n142 = call "Manual Controls Action Engine.vi"("Action"=enum16{"Read", "Write"}."Read") -> ("Manual Controls Out"=w198:T17)  [unwired: 14 in]
            n143 = Bundle By Name(cluster=w198, "Res Mirror Amp (I16)"=w204, "Res Mirror Mute"=w190) -> (w196:T17)
            n144 = call "Image Aquisition Param Ctrl_AE.vi"("Action"=enum16{"READ", "WRITE"}."WRITE", "Image Acquisition Parameters In"=w192) -> ()  [unwired: 9 in, 1 out]
            n145 = call "FPGA-7842R-Control V1.vi"("Action"=FPGA-7842R-Reference."Set Res Mirror", "Manual Controls"=w196, "Initialize"=TRUE) -> ()  [unwired: 11 in, 2 out]
            n146 = call "Manual Controls Action Engine.vi"("Action"=enum16{"Read", "Write"}."Write", "Manual Controls In"=w196) -> ()  [unwired: 13 in, 1 out]
          }
          frame "Detectors" {
            n147 = call "Detectors Crl_AE.vi"("Action"=enum16{"READ", "WRITE"}."WRITE", "Detectors Parameters In"="Detectors") -> ()  [unwired: 9 in, 1 out]
          }
          frame "Laser Controls" {
            w253 = FALSE ("element")
            n148 = Unbundle By Name("Laser Controls") -> ("STED"=w259:bool, "640 nm"=w256:bool, "590 nm"=w257:bool, "485 nm"=w258:bool, "STED Power (V)"=w250:dbl, "Manual Control"=w244:bool)
            n149 = local read "Live"() -> (w245:bool)
            n150 = call "LASERs_ Crl_AE.vi"("Action"=enum16{"READ", "WRITE"}."WRITE", "Detectors Parameters In"="Laser Controls") -> ()  [unwired: 9 in, 1 out]
            n151 = Or(x=w245, y=w244) -> (x .or. y?=w243:bool)
            n152 = In Range and Coerce(upper limit=10.0, x=w250, lower limit=0.0) -> (coerced(x)=w247:dbl)  [unwired: 1 out]
            n153 = Build Array(w259, w256, w257, w258, w253, w253, w253, w253) -> (w255:bool[])
            n154 = case shown="True" w243 {
              tunnel: "Laser Controls" -> [_ w265]
              frame False {
              }
              frame True {
                n155 = call "FPGA-7842R-Control V1.vi"("Action"=FPGA-7842R-Reference."Laser Control", "Laser Controls"=w265, "Initialize"=TRUE) -> ()  [unwired: 11 in, 2 out]
              }
            }
            n156 = Boolean Array To Number(Boolean array=w255) -> (number=w254:u32)
            n157 = To Unsigned Byte Integer(number=w254) -> (unsigned 8bit integer=w252:u8)
            n158 = call "U8_To_U32.vi"("U8 IN"=w252) -> ("U32 OUT"=w251:u32)  [unwired: 13 in, 1 out]
            n159 = call "Volts to I16.vi"("Voltage (V)"=w247) -> ("I16"=w246:i16)  [unwired: 13 in, 1 out]
            n160 = call "Scan Parameters Action Engine.vi"("Action"=enum16{"Read", "Write"}."Read") -> ("Scan Parameters OUT"=w262:T16)  [unwired: 14 in]
            n161 = Bundle By Name(cluster=w262, "Laser_States _U32"=w251, "775_AOM_Volt_I16"=w246) -> (w260:T16)
            n162 = call "Scan Parameters Action Engine.vi"("Action"=enum16{"Read", "Write"}."Write", "Scan Parameters IN"=w260) -> ()  [unwired: 13 in, 1 out]
          }
          frame "Shutters" {
            n163 = Unbundle By Name("Shutters") -> ("Upper Shutter"=w277:bool, "Lower Shutter"=w276:bool)
            n164 = Not(x=w277) -> (.not. x?=w268:bool)
            n165 = Not(x=w276) -> (.not. x?=w267:bool)
            n166 = call "Manual Controls Action Engine.vi"("Action"=enum16{"Read", "Write"}."Read") -> ("Manual Controls Out"=w272:T17)  [unwired: 14 in]
            n167 = Bundle By Name(cluster=w272, "Upper Shutter"=w268, "Lower Shutter"=w267) -> (w269:T17)
            n168 = call "Manual Controls Action Engine.vi"("Action"=enum16{"Read", "Write"}."Write", "Manual Controls In"=w269) -> ()  [unwired: 13 in, 1 out]
            n169 = call "FPGA-7842R-Control V1.vi"("Action"=FPGA-7842R-Reference."Shutter Control", "Manual Controls"=w269, "Initialize"=TRUE) -> ()  [unwired: 11 in, 2 out]
          }
        }
      }
      event Value Change {
        # "For P541 - Sample Z - Converting from Step in µm to I16 is as follows. We have (Step µw)*(10 V / 100 µm)*(32768 I16 / 10 V) = (Step µm)*(32768 I16 / 100 µm) = (Step µm)*(327.68 I16/µm)"
        n170 = event-data() -> ("CtlRef"=w291:refnum<vi>, "OldVal"=w289:variant, "NewVal"=w290:variant)  [unwired: 1 in]
        n171 = local write "Abort AllStage"(FALSE ("Abort AllStage")) -> ()
        n172 = property class="Clust"(reference=w291) -> ("Label.Text"=w288:string)  [unwired: 1 in, 2 out]
        n173 = case shown="Default" w288 {
          tunnel: w290 -> [_ w314 w342 w369 w432 w459 w485]
          tunnel: w289 -> [_ w313 w341 w368 w433 w460 w486]
          tunnel: ["" "N664" "ASI" "P612" "P612" "P841" "M227"] -> w287
          tunnel: [dbl[] [0.0] w305 w334 w357 dbl[] [0.0] w448 w475] -> w286
          tunnel: [bool[] [FALSE] w303 w328 w358 bool[] [FALSE] bool[] [TRUE] w477] -> w285
          tunnel: [enum16{"MOVE", "MVR"}."MVR" ("MOVE/MVR") w302 w331 w360 enum16{"MOVE", "MVR"}."MVR" ("MOVE/MVR") w451 enum16{"MOVE", "MVR"}."MVR" ("MOVE/MVR")] -> w284
          tunnel: [0.0 ("Step Size (um)") 0.5 ("Step Size (um)") w333 0.0 ("Velocity") 0.0 ("Velocity") 10000.0 ("Velocity") 0.0 ("Velocity")] -> w280
          tunnel: [StageStates."MVR" ("Action") w300 w332 w361 StageStates."POSITION" ("Action") w452 StageStates."MVR" ("Action")] -> w278
          frame Default {
          }
          frame "Upper Objective Z - N664" {
            n174 = call "N664_Ctrl_Index.vi"("OldVal"=w313, "NewVal"=w314) -> ("Control Ref OUT"=w312:refnum<vi>, "N664 Out"=w310:T4)  [unwired: 12 in]
            n175 = property class="Ctl"(reference=w312) -> ("Label.Text"=w311:string)  [unwired: 1 in, 2 out]
            n176 = Unbundle By Name(w310) -> ("Step Size (um)"=w309:dbl, "Position (mm)"=w308:dbl)
            n177 = case shown="\"Down N664\"" w311 {
              tunnel: w309 -> [_ w320 w324 _]
              tunnel: [0.0 ("Step Size (um)") w320 w323 w327] -> w306
              tunnel: w308 -> [_ _ _ w327]
              tunnel: [enum16{"MOVE", "MVR"}."MVR" ("MOVE/MVR") enum16{"MOVE", "MVR"}."MVR" ("MOVE/MVR") enum16{"MOVE", "MVR"}."MVR" ("MOVE/MVR") enum16{"MOVE", "MVR"}."MOVE" ("MOVE/MVR")] -> w302
              tunnel: [StageStates."MVR" ("Action") StageStates."MVR" ("Action") StageStates."MVR" ("Action") StageStates."MOVE" ("Action")] -> w300
              frame Default {
              }
              frame "Up N664" {
              }
              frame "Down N664" {
                n178 = Negate(x=w324) -> (-x=w323:dbl)
              }
              frame "Position (mm)" {
              }
            }
            n179 = Build Array(w306) -> (w305:dbl[])
            n180 = Build Array(TRUE) -> (w303:bool[])
          }
          frame "Cavity Translation Z - ASI" {
            n181 = call "ASI_Ctrl_Index.vi"("NewVal"=w342, "OldVal"=w341) -> ("ASI out"=w338:T5, "Control Ref OUT"=w340:refnum<vi>)  [unwired: 8 in]
            n182 = property class="Ctl"(reference=w340) -> ("Label.Text"=w339:string)  [unwired: 1 in, 2 out]
            n183 = Unbundle By Name(w338) -> ("Step Size (um)"=w337:dbl, "Z (um)"=w336:dbl, "Velocity"=w333:dbl)
            n184 = case shown="\"Down ASI\"" w339 {
              tunnel: w337 -> [_ w348 w351 _]
              tunnel: w336 -> [_ _ _ w355]
              tunnel: [0.0 ("Z (um)") w348 w352 w355] -> w335
              tunnel: [StageStates."MVR" ("Action") StageStates."MVR" ("Action") StageStates."MVR" ("Action") StageStates."MOVE" ("Action")] -> w332
              tunnel: [enum16{"MOVE", "MVR"}."MVR" ("MOVE/MVR") enum16{"MOVE", "MVR"}."MVR" ("MOVE/MVR") enum16{"MOVE", "MVR"}."MVR" ("MOVE/MVR") enum16{"MOVE", "MVR"}."MOVE" ("MOVE/MVR")] -> w331
              frame Default {
              }
              frame "Up ASI" {
              }
              frame "Down ASI" {
                n185 = Negate(x=w351) -> (-x=w352:dbl)
              }
              frame "Z (um)" {
              }
            }
            n186 = Build Array(w335) -> (w334:dbl[])
            n187 = Build Array(TRUE) -> (w328:bool[])
          }
          frame "Bottom Objective XY - P612" {
            n188 = call "P612_Ctrl_Index.vi"("OldVal"=w368, "NewVal"=w369) -> ("Control out"=w367:refnum<vi>, "P612 out"=w365:T8)  [unwired: 12 in]
            n189 = property class="Ctl"(reference=w367) -> ("Label.Text"=w366:string)  [unwired: 1 in, 2 out]
            n190 = Unbundle By Name(w365) -> ("Step Size (um)"=w364:dbl, "X"=w363:dbl, "Y"=w362:dbl)
            n191 = case shown="\"Up Button\"" w366 {
              tunnel: w364 -> [_ _ w380 w387 w391 w398 _]
              tunnel: w363 -> [_ _ _ _ _ _ w405]
              tunnel: w362 -> [_ _ _ _ _ _ w404]
              tunnel: [StageStates."MVR" ("Action") StageStates."HOME" ("Action") StageStates."MVR" ("Action") StageStates."MVR" ("Action") StageStates."MVR" ("Action") StageStates."MVR" ("Action") StageStates."MOVE" ("Action")] -> w361
              tunnel: [enum16{"MOVE", "MVR"}."MVR" ("MOVE/MVR") enum16{"MOVE", "MVR"}."MVR" ("MOVE/MVR") enum16{"MOVE", "MVR"}."MVR" ("MOVE/MVR") enum16{"MOVE", "MVR"}."MVR" ("MOVE/MVR") enum16{"MOVE", "MVR"}."MVR" ("MOVE/MVR") enum16{"MOVE", "MVR"}."MVR" ("MOVE/MVR") enum16{"MOVE", "MVR"}."MOVE" ("MOVE/MVR")] -> w360
              tunnel: [bool[] [FALSE] bool[] [TRUE, TRUE] bool[] [TRUE, FALSE] bool[] [TRUE, FALSE] bool[] [FALSE, TRUE] bool[] [FALSE, TRUE] bool[] [TRUE, TRUE]] -> w358
              tunnel: [dbl[] [0.0] dbl[] [0.0, 0.0] w379 w386 w393 w400 w406] -> w357
              frame Default {
              }
              frame "Home Button" {
              }
              frame "Up Button" {
                n192 = Build Array(w380, 0.0 ("element")) -> (w379:dbl[])
              }
              frame "Down Button" {
                n193 = Negate(x=w387) -> (-x=w384:dbl)
                n194 = Build Array(w384, 0.0 ("element")) -> (w386:dbl[])
              }
              frame "Left Button" {
                n195 = Build Array(0.0 ("element"), w391) -> (w393:dbl[])
              }
              frame "Right Button" {
                n196 = Negate(x=w398) -> (-x=w397:dbl)
                n197 = Build Array(0.0 ("element"), w397) -> (w400:dbl[])
              }
              frame "X", "Y" {
                n198 = Build Array(w405, w404) -> (w406:dbl[])
              }
            }
          }
          frame "Sample Z - P541" {
            w425 = 327.68 ("y")
            n199 = call "P541_Ctrl_Index.vi"("OldVal"=w433, "NewVal"=w432) -> ("Control out"=w431:refnum<vi>, "P541 Out"=w430:T12)  [unwired: 12 in]
            n200 = property class="Ctl"(reference=w431) -> ("Label.Text"=w428:string)  [unwired: 1 in, 2 out]
            n201 = Unbundle By Name(w430) -> ("Z Position"=w426:dbl, "Step Size (um)"=w429:dbl)
            n202 = call "Manual Controls Action Engine.vi"("Action"=enum16{"Read", "Write"}."Read") -> ("Manual Controls Out"=w417:T17)  [unwired: 14 in]
            n203 = Unbundle By Name(w417) -> ("Z Axis Voltage (I16)"=w420:i16)
            n204 = Multiply(x=w425, y=w426) -> (x*y=w423:dbl)
            n205 = Multiply(x=w429, y=w425) -> (x*y=w427:dbl)
            n206 = Round To Nearest(number=w423) -> (nearest integer value=w412:dbl)
            n207 = Round To Nearest(number=w427) -> (nearest integer value=w411:dbl)
            n208 = To Word Integer(number=w412) -> (16bit integer=w422:i16)
            n209 = To Word Integer(number=w411) -> (16bit integer=w424:i16)
            n210 = case shown="\"Step Down\"" w428 {
              tunnel: w424 -> [_ w440 w444 _]
              tunnel: w422 -> [_ _ _ w446]
              tunnel: w420 -> [w439 w442 w445 _]
              tunnel: [w439 w441 w443 w446] -> w416
              frame Default {
              }
              frame "Step Down" {
                n211 = Subtract(x=w442, y=w440) -> (x-y=w441:i16)
              }
              frame "Step Up" {
                n212 = Add(x=w445, y=w444) -> (x+y=w443:i16)
              }
              frame "Z Position" {
              }
            }
            n213 = Bundle By Name(cluster=w417, "Z Axis Voltage (I16)"=w416) -> (w419:T17)
            n214 = call "Manual Controls Action Engine.vi"("Action"=enum16{"Read", "Write"}."Write", "Manual Controls In"=w419) -> ("Manual Controls Out"=w413:T17)  [unwired: 13 in]
            n215 = call "FPGA-7842R-Control V1.vi"("Action"=FPGA-7842R-Reference."Stage Control", "Manual Controls"=w413, "Initialize"=TRUE) -> ()  [unwired: 11 in, 2 out]
          }
          frame "Phase Comp Mirror - P841" {
            n216 = call "P841_Ctrl_Index.vi"("OldVal"=w460, "NewVal"=w459) -> ("Control out"=w457:refnum<vi>, "P841 Out"=w455:T6)  [unwired: 12 in]
            n217 = property class="Ctl"(reference=w457) -> ("Label.Text"=w456:string)  [unwired: 1 in, 2 out]
            n218 = Unbundle By Name(w455) -> ("Position (µm)"=w454:dbl, "Step Size (µm)"=w453:dbl)
            n219 = case shown="\"Down P841\"" w456 {
              tunnel: w454 -> [_ _ _ w473]
              tunnel: w453 -> [_ w466 w470 _]
              tunnel: [0.0 ("Position (µm)") w466 w469 w473] -> w449
              tunnel: [StageStates."MVR" ("Action") StageStates."MVR" ("Action") StageStates."MVR" ("Action") StageStates."MOVE" ("Action")] -> w452
              tunnel: [enum16{"MOVE", "MVR"}."MVR" ("MOVE/MVR") enum16{"MOVE", "MVR"}."MVR" ("MOVE/MVR") enum16{"MOVE", "MVR"}."MVR" ("MOVE/MVR") enum16{"MOVE", "MVR"}."MOVE" ("MOVE/MVR")] -> w451
              frame Default {
              }
              frame "Up P841" {
              }
              frame "Down P841" {
                n220 = Negate(x=w470) -> (-x=w469:dbl)
              }
              frame "Position (µm)" {
              }
            }
            n221 = Build Array(w449) -> (w448:dbl[])
          }
          frame "Sample Z Coarse - M227" {
            n222 = call "M227_Ctrl_Index.vi"("OldVal"=w486, "NewVal"=w485) -> ("Control Ref OUT"=w484:refnum<vi>, "M227 Out"=w482:T10)  [unwired: 12 in]
            n223 = property class="Ctl"(reference=w484) -> ("Label.Text"=w483:string)  [unwired: 1 in, 2 out]
            n224 = Unbundle By Name(w482) -> ("Step Size (mm)"=w481:dbl)
            n225 = case shown="\"Down M227\"" w483 {
              tunnel: w481 -> [_ w489 w492]
              tunnel: [bool[] [FALSE, FALSE, FALSE] bool[] [TRUE, TRUE, TRUE] bool[] [TRUE, TRUE, TRUE]] -> w477
              tunnel: [0.0 ("Step Size (mm)") w489 w491] -> w476
              frame Default {
              }
              frame "Up M227" {
              }
              frame "Down M227" {
                n226 = Negate(x=w492) -> (-x=w491:dbl)
              }
            }
            n227 = Build Array(w476) -> (w475:dbl[])
          }
        }
        n228 = case shown="\"Upper Objective Z - N664\"" w288 {
          frame Default {
          }
          frame "Upper Objective Z - N664" {
            n229 = while {
              i -> [w498]
              stop <- w494 stop-if-true
              n230 = call "Stage_position_ae.vi"("StageID"="N664", "Enum"=enum16{"WRITE", "READ"}."READ") -> ("Status Out"=w495:bool, "Position Out"=w506:dbl[])  [unwired: 8 in]
              n231 = Greater?(x=w498, y=200) -> (0:w497:bool)
              n232 = And(x=w495, y=w497) -> (x .and. y?=w494:bool)
              n233 = Wait (ms)(milliseconds to wait=u32 1) -> ()  [unwired: 1 out]
              n234 = Index Array(array=w506, index=0) -> (element=w505:dbl)
              n235 = Select(t=u32 16777215, s=w494, f=u32 6618880) -> (s? t:f=w499:u32)
              n236 = property on="Position (mm)" class="DigNum (strict)"("Value"=w505, "NumText.BG Color"=w499) -> ()  [unwired: 2 in, 2 out]
            }
          }
          frame "Cavity Translation Z - ASI" {
            n237 = while {
              shift-right: [w509] -> _
              shift-left: TRUE ("Status Out") -> [w514]
              stop <- w513 stop-if-true
              n238 = call "Stage_position_ae.vi"("StageID"="ASI", "Enum"=enum16{"WRITE", "READ"}."READ") -> ("Status Out"=w509:bool, "Position Out"=w519:dbl[])  [unwired: 8 in]
              n239 = Greater?(x=w509, y=w514) -> (0:w513:bool)
              n240 = Wait (ms)(milliseconds to wait=u32 1) -> ()  [unwired: 1 out]
              n241 = Index Array(array=w519, index=0) -> (element=w518:dbl)
              n242 = Select(t=u32 16777215, s=w509, f=u32 6618880) -> (s? t:f=w510:u32)
              n243 = property on="Z (um)" class="DigNum (strict)"("Value"=w518, "NumText.BG Color"=w510) -> ()  [unwired: 2 in, 2 out]
            }
          }
        }
        n244 = control-ref of="Abort AllStage"() -> (w279:refnum<vi>)
        n245 = call "AllStage_Limits_Array.vi"("Step(um)/Position(units)"=w286, "Axis"=w285, "Stage ID"=w287, "MOVE/MVR"=w284) -> ("Positions"=w282:dbl[], "Boolean Array"=w281:bool[], "Stage ID"=w283:string)  [unwired: 5 in]
        n246 = call "AE_AllStages_Action V2.vi"("Velocity"=w280, "Abort"=w279, "Positions"=w282, "Axis"=w281, "Stage ID"=w283, "Action"=w278) -> ()  [unwired: 3 in, 3 out]
      }
      event "SLM", "Timing", "DM": Value Change {
        n247 = event-data() -> ("CtlRef"=w524:refnum<vi>, "NewVal"=w521:bool)  [unwired: 1 in, 1 out]
        n248 = property class="Bool (strict)"(reference=w524) -> ("Label.Text"=w523:string)  [unwired: 1 in, 2 out]
        n249 = case shown="\"SLM\", Default" w523 {
          tunnel: w521 -> [w525 w539 w553]
          frame "SLM", Default {
            n250 = case shown="False" w525 {
              frame False {
                n251 = To Variant(anything=TRUE) -> (Variant=w531:variant)
                n252 = call "SLM AE.vi"("Action"=enum16{"READ", "WRITE"}."READ") -> ("SLM Ref Out"=w532:refnum<vi>)  [unwired: 10 in]
                n253 = invoke class="VI" method="Ctrl Val.Set"(reference=w532, "Control Name"="Exit", "Value"=w531) -> (reference out=w528:refnum<vi>, error out=w527:errorcluster)  [unwired: 2 in, 3 out]
                n254 = invoke on="Hamamatsu LCOS" class="SubPnl" method="Remove VI"(error in=w527) -> (error out=w526:errorcluster)  [unwired: 2 in, 2 out]
                n255 = Close Reference(reference=w528, error in (no error)=w526) -> ()  [unwired: 1 out]
              }
              frame True {
                n256 = Open VI Reference(vi path=path "C:/Users/ED STED/Documents/Test Control Software/Host VIs/SLM/SLM Control.vi") -> (vi reference=w537:refnum<vi>)  [unwired: 5 in, 1 out]
                n257 = invoke class="VI" method="Run VI"(reference=w537, "Wait until done"=FALSE ("Wait Until Done")) -> (reference out=w534:refnum<vi>)  [unwired: 3 in, 4 out]
                n258 = invoke on="Hamamatsu LCOS" class="SubPanel" method="Insert VI"("VI Ref"=w534) -> ()  [unwired: 3 in, 4 out]
                n259 = call "SLM AE.vi"("Action"=enum16{"READ", "WRITE"}."WRITE", "SLM Ref In"=w534) -> ()  [unwired: 9 in, 1 out]
              }
            }
          }
          frame "DM" {
            n260 = case shown="True" w539 {
              frame False {
                n261 = call "DM_Ref_AE.vi"("Action"=enum16{"READ", "WRITE"}."READ") -> ("DM Ref Out"=w546:refnum<vi>)  [unwired: 10 in]
                n262 = To Variant(anything=TRUE) -> (Variant=w545:variant)
                n263 = invoke class="VI" method="Ctrl Val.Set"(reference=w546, "Control Name"="Exit", "Value"=w545) -> (reference out=w542:refnum<vi>, error out=w541:errorcluster)  [unwired: 2 in, 3 out]
                n264 = invoke on="Hamamatsu LCOS" class="SubPnl" method="Remove VI"(error in=w541) -> (error out=w540:errorcluster)  [unwired: 2 in, 2 out]
                n265 = Close Reference(reference=w542, error in (no error)=w540) -> ()  [unwired: 1 out]
              }
              frame True {
                n266 = Open VI Reference(vi path=path "C:/Users/ED STED/Documents/Test Control Software/Host VIs/DM/DM_Control_STED.vi") -> (vi reference=w551:refnum<vi>)  [unwired: 5 in, 1 out]
                n267 = invoke class="VI" method="Run VI"(reference=w551, "Wait until done"=FALSE ("Wait Until Done")) -> (reference out=w548:refnum<vi>)  [unwired: 3 in, 4 out]
                n268 = invoke on="BM Multi" class="SubPanel" method="Insert VI"("VI Ref"=w548) -> ()  [unwired: 3 in, 4 out]
                n269 = call "DM_Ref_AE.vi"("Action"=enum16{"READ", "WRITE"}."WRITE", "DM Ref In"=w548) -> ()  [unwired: 9 in, 1 out]
              }
            }
          }
          frame "Timing" {
            n270 = case shown="True" w553 {
              frame False {
                n271 = To Variant(anything=TRUE) -> (Variant=w558:variant)
                n272 = call "GateDelay AE.vi"("Action"=enum16{"READ", "WRITE"}."READ") -> ("Gate Delay Ref Out"=w559:refnum<vi>)  [unwired: 10 in]
                n273 = invoke class="VI" method="Ctrl Val.Set"(reference=w559, "Control Name"="Exit", "Value"=w558) -> (reference out=w554:refnum<vi>, error out=w555:errorcluster)  [unwired: 2 in, 3 out]
                n274 = invoke on="Timing" class="SubPnl" method="Remove VI"(error in=w555) -> (error out=w561:errorcluster)  [unwired: 2 in, 2 out]
                n275 = Close Reference(reference=w554, error in (no error)=w561) -> ()  [unwired: 1 out]
              }
              frame True {
                n276 = Open VI Reference(vi path=path "C:/Users/ED STED/Documents/Test Control Software/Host VIs/Time Delay/GateDelay_Control_V1.vi") -> (vi reference=w564:refnum<vi>)  [unwired: 5 in, 1 out]
                n277 = invoke class="VI" method="Run VI"(reference=w564, "Wait until done"=FALSE ("Wait Until Done")) -> (reference out=w563:refnum<vi>)  [unwired: 3 in, 4 out]
                n278 = invoke on="Timing" class="SubPanel" method="Insert VI"("VI Ref"=w563) -> ()  [unwired: 3 in, 4 out]
                n279 = call "GateDelay AE.vi"("Action"=enum16{"READ", "WRITE"}."WRITE", "Gate Delay Ref In"=w563) -> ()  [unwired: 9 in, 1 out]
              }
            }
          }
        }
      }
      event Value Change {
        n280 = event-data() -> ("CtlRef"=w572:refnum<vi>, "OldVal"=w570:variant, "NewVal"=w569:variant)  [unwired: 1 in]
        n281 = property class="Clust"(reference=w572) -> ("Label.Text"=w571:string)  [unwired: 1 in, 2 out]
        n282 = call "Graph Ref AE.vi"("Action"=enum16{"READ", "WRITE"}."READ") -> ("Graph Ref Out"=w567:refnum<vi>[])  [unwired: 10 in]
        n283 = case shown="\"Display Controls\"" w571 {
          tunnel: w570 -> [_ w579 w635]
          tunnel: w569 -> [_ w580 w634]
          tunnel: w567 -> [_ w574 w627]
          frame Default {
          }
          frame "Display Controls" {
            n284 = call "Display_Controls_Ctrl_Index.vi"("OldVal"=w579, "NewVal"=w580) -> ("Control Ref OUT"=w578:refnum<vi>, "Display Controls Out"=w576:T1)  [unwired: 12 in]
            n285 = property class="Ctl"(reference=w578) -> ("Label.Text"=w577:string)  [unwired: 1 in, 2 out]
            n286 = Unbundle By Name(w576) -> ("Single Screen"=w575:bool)
            n287 = case shown="\"Single Screen\", Default" w577 {
              tunnel: w575 -> [w588 _ _]
              tunnel: w574 -> [_ w613 w620]
              frame "Single Screen", Default {
                n288 = property class="App"() -> ("Disp.AllMonitors"=w587:T30)  [unwired: 2 in, 2 out]
                n289 = Index Array(array=w587, index #1=2 ("index"), index #2=0 ("index")) -> (element #1=w584:T31, element #2=w583:T31)
                n290 = control-ref of="This VI"() -> (w582:refnum<vi>)
                n291 = case shown="False" w588 {
                  tunnel: w584 -> [w592 _]
                  tunnel: w583 -> [w591 w603]
                  tunnel: w582 -> [w590 w601]
                  tunnel: T21 {"Left"=0, "Top"=0, "Right"=0, "Bottom"=0} ("Front Panel Window:Window Bounds") -> [w589 w602]
                  frame False {
                    w597 = i16 0
                    n292 = Unbundle By Name(w591) -> ("Bounds.Left"=w594:i16, "Bounds.Bottom"=w595:i16, "Bounds.Top"=w596:i16)
                    n293 = Unbundle By Name(w592) -> ("Bounds.Right"=w593:i16)
                    n294 = Subtract(x=w593, y=w594) -> (x-y=w598:i16)
                    n295 = Subtract(x=w595, y=w596) -> (x-y=w599:i16)
                    n296 = Bundle By Name(cluster=w589, "Left"=w597, "Top"=w597, "Right"=w598, "Bottom"=w599) -> (w600:T21)
                    n297 = property class="VI"(reference=w590, "Front Panel.WinBounds"=w600) -> ()  [unwired: 1 in, 2 out]
                  }
                  frame True {
                    w606 = i16 0
                    n298 = Unbundle By Name(w603) -> ("Bounds.Right"=w609:i16, "Bounds.Bottom"=w608:i16, "Bounds.Top"=w607:i16)
                    n299 = Subtract(x=w608, y=w607) -> (x-y=w605:i16)
                    n300 = Bundle By Name(cluster=w602, "Left"=w606, "Top"=w606, "Right"=w609, "Bottom"=w605) -> (w604:T21)
                    n301 = property class="VI"(reference=w601, "Front Panel.WinBounds"=w604) -> (reference out=w611:refnum<vi>)  [unwired: 1 in, 1 out]
                    n302 = property class="VI"(reference=w611, "FP.State"=T22."Maximized" ("Front Panel Window:State")) -> ()  [unwired: 1 in, 2 out]
                  }
                }
              }
              frame "Add Display" {
                w614 = u16 0 items=["Read", "Write"] ("Action")
                w618 = u16 1 items=["Read", "Write"] ("Action")
                n303 = property on="Add Display" class="Bool (strict)"("Value"=FALSE) -> ()  [unwired: 2 in, 2 out]
                n304 = call "Arange_Displays_V2.vi"("Action"=w614) -> ("Number of Channels OUT"=w615:i32)  [unwired: 14 in]
                n305 = Increment(x=w615) -> (x+1=w617:i32)
                n306 = call "Arange_Displays_V2.vi"("Display References"=w613, "Action"=w618, "Number of Channels"=w617, "Aspect Ratio (h/w)"=1.0) -> ()  [unwired: 11 in, 1 out]
              }
              frame "Remove Display" {
                w621 = u16 0 items=["Read", "Write"] ("Action")
                w625 = u16 1 items=["Read", "Write"] ("Action")
                n307 = call "Arange_Displays_V2.vi"("Action"=w621) -> ("Number of Channels OUT"=w622:i32)  [unwired: 14 in]
                n308 = Decrement(x=w622) -> (x-1=w624:i32)
                n309 = call "Arange_Displays_V2.vi"("Display References"=w620, "Action"=w625, "Number of Channels"=w624, "Aspect Ratio (h/w)"=1.0) -> ()  [unwired: 11 in, 1 out]
                n310 = property on="Remove Display" class="Bool (strict)"("Value"=FALSE) -> ()  [unwired: 2 in, 2 out]
              }
            }
          }
          frame "Graph Tools" {
            n311 = call "Graph_Controls_Ctrl_Index.vi"("OldVal"=w635, "NewVal"=w634) -> ("Control Ref OUT"=w633:refnum<vi>, "Graph Tools Out"=w632:T2)  [unwired: 12 in]
            n312 = property class="Ctl"(reference=w633) -> (reference out=w629:refnum<vi>, "Label.Text"=w628:string)  [unwired: 1 in, 1 out]
            n313 = Unbundle By Name(w632) -> ("Show Cursor"=w631:bool, "Auto Scale"=w630:bool, "Color Map"=w626:T32)
            n314 = case shown="\"Apply Color\"" w628 {
              selector: w628 -> [_ _ _ w704 _ _ _ _]
              tunnel: w631 -> [_ w673 _ _ _ _ _ _]
              tunnel: w630 -> [_ _ w693 _ _ _ _ _]
              tunnel: w627 -> [w644 w672 w694 w697 w734 _ w746 w754]
              tunnel: w629 -> [_ _ _ _ _ _ _ _]
              tunnel: w628 -> [_ _ _ w699 _ _ _ _]
              tunnel: w626 -> [w647 _ _ _ _ _ _ _]
              frame "Apply Color" {
                n315 = control-ref of="This VI"() -> (w646:refnum<vi>)
                n316 = call "GetDisplayClick.vi"("Display REFs In"=w644, "Calling VI REF"=w646) -> ("Display Index"=w645:i32)  [unwired: 13 in]
                n317 = Index Array(array=w644, index=w645) -> (element=w643:refnum<vi>)
                n318 = property class="IntGraph (strict)"(reference=w643) -> (reference out=w639:refnum<vi>, error out=w636:errorcluster, "ZScale.Maximum"=w642:dbl)  [unwired: 1 in]
                n319 = case shown="\"Fire\", Default" w647 {
                  tunnel: [cluster{dbl, u32}[] [{0.0, 0}, {85.0, 16711680}, {108.0, 16729344}, {127.0, 16744192}, {132.0, 16747520}, {140.0, 16753920}, {157.0, 16766720}, {170.0, 16776960}, {245.0, 16777184}, {250.0, 16777200}, {255.0, 16777215}] ("Z Scale.Marker Values[]") cluster{dbl, u32}[] [{0.0, 0}, {255.0, 16777215}] ("Z Scale.Marker Values[]") cluster{dbl, u32}[] [{0.0, 0}, {255.0, 16711680}] ("Z Scale.Marker Values[]") cluster{dbl, u32}[] [{0.0, 0}, {255.0, 65280}] ("Z Scale.Marker Values[]") cluster{dbl, u32}[] [{0.0, 0}, {255.0, 255}] ("Z Scale.Marker Values[]") cluster{dbl, u32}[] [{0.0, 0}, {255.0, 65535}] ("Z Scale.Marker Values[]") cluster{dbl, u32}[] [{0.0, 0}, {255.0, 16711935}] ("Z Scale.Marker Values[]") cluster{dbl, u32}[] [{0.0, 0}, {255.0, 16776960}] ("Z Scale.Marker Values[]") cluster{dbl, u32}[] [{0.0, 0}, {170.0, 16711680}, {245.0, 16777184}, {250.0, 16777200}, {255.0, 16448250}] ("Z Scale.Marker Values[]") cluster{dbl, u32}[] [{0.0, 0}, {170.0, 65280}, {245.0, 16777184}, {250.0, 16777200}, {255.0, 16448250}] ("Z Scale.Marker Values[]") cluster{dbl, u32}[] [{0.0, 0}, {170.0, 255}, {245.0, 16777184}, {250.0, 16777200}, {255.0, 16448250}] ("Z Scale.Marker Values[]") cluster{dbl, u32}[] [{0.0, 0}, {1.0, 131072}, {2.0, 196608}, {3.0, 327680}, {4.0, 458752}, {5.0, 589824}, {6.0, 720896}, {7.0, 851971}, {8.0, 983043}, {9.0, 1114115}, {10.0, 1245187}, {11.0, 1376259}, {12.0, 1507331}, {13.0, 1638403}, {14.0, 1769475}, {15.0, 1769479}, {16.0, 2031623}, {17.0, 2162695}, {18.0, 2293767}, {19.0, 2424839}, {20.0, 2555911}, {21.0, 2686983}, {22.0, 2818055}, {23.0, 2949127}, {24.0, 3080203}, {25.0, 3211275}, {26.0, 3342347}, {27.0, 3473419}, {28.0, 3604491}, {29.0, 3735563}, {30.0, 3866635}, {31.0, 3867403}, {32.0, 4129547}, {33.0, 4260619}, {34.0, 4391691}, {35.0, 4522763}, {36.0, 4653839}, {37.0, 4784911}, {38.0, 4915983}, {39.0, 5178127}, {40.0, 5309199}, {41.0, 5440271}, {42.0, 5571343}, {43.0, 5702415}, {44.0, 5703439}, {45.0, 5965583}, {46.0, 6096655}, {47.0, 6227727}, {48.0, 6358799}, {49.0, 6489871}, {50.0, 6620943}, {51.0, 6752015}, {52.0, 6883087}, {53.0, 7015183}, {54.0, 7146255}, {55.0, 7277327}, {56.0, 7408399}, {57.0, 7539471}, {58.0, 7670543}, {59.0, 7801615}, {60.0, 8063759}, {61.0, 8194831}, {62.0, 8326927}, {63.0, 8457999}, {64.0, 8589075}, {65.0, 8720147}, {66.0, 8851219}, {67.0, 8982291}, {68.0, 9113363}, {69.0, 9114387}, {70.0, 9376531}, {71.0, 9507603}, {72.0, 9638675}, {73.0, 9769747}, {74.0, 9901843}, {75.0, 10032915}, {76.0, 10163987}, {77.0, 10229523}, {78.0, 10295059}, {79.0, 10427155}, {80.0, 10558227}, {81.0, 10689299}, {82.0, 10820371}, {83.0, 10886931}, {84.0, 10952467}, {85.0, 11083539}, {86.0, 11214611}, {87.0, 11215635}, {88.0, 11477779}, {89.0, 11543315}, {90.0, 11608851}, {91.0, 11740947}, {92.0, 11806483}, {93.0, 11872019}, {94.0, 12004115}, {95.0, 12135187}, {96.0, 12266259}, {97.0, 12267283}, {98.0, 12398355}, {99.0, 12529427}, {100.0, 12530451}, {101.0, 12595987}, {102.0, 12530451}, {103.0, 12793619}, {104.0, 12794131}, {105.0, 12794643}, {106.0, 13056787}, {107.0, 13057299}, {108.0, 13057811}, {109.0, 13188883}, {110.0, 13320979}, {111.0, 13386515}, {112.0, 13452563}, {113.0, 13584147}, {114.0, 13584659}, {115.0, 13585171}, {116.0, 13585683}, {117.0, 13717267}, {118.0, 13848339}, {119.0, 13849363}, {120.0, 13849875}, {121.0, 13850387}, {122.0, 13981459}, {123.0, 14113555}, {124.0, 14114067}, {125.0, 14114579}, {126.0, 14115091}, {127.0, 14246675}, {128.0, 14377747}, {129.0, 14378771}, {130.0, 14379283}, {131.0, 14379539}, {132.0, 14379795}, {133.0, 14380819}, {134.0, 14511891}, {135.0, 14643987}, {136.0, 14644503}, {137.0, 14645015}, {138.0, 14645527}, {139.0, 14646039}, {140.0, 14646551}, {141.0, 14778135}, {142.0, 14909207}, {143.0, 14910231}, {144.0, 14910747}, {145.0, 14911259}, {146.0, 14911771}, {147.0, 14912283}, {148.0, 14912797}, {149.0, 15044383}, {150.0, 15175455}, {151.0, 15175967}, {152.0, 15176479}, {153.0, 15176991}, {154.0, 15177507}, {155.0, 15178019}, {156.0, 15178531}, {157.0, 15310115}, {158.0, 15441701}, {159.0, 15441959}, {160.0, 15442215}, {161.0, 15442727}, {162.0, 15443243}, {163.0, 15443755}, {164.0, 15444269}, {165.0, 15444783}, {166.0, 15444783}, {167.0, 15576367}, {168.0, 15707953}, {169.0, 15708467}, {170.0, 15708979}, {171.0, 15708981}, {172.0, 15708983}, {173.0, 15710011}, {174.0, 15710523}, {175.0, 15711037}, {176.0, 15711039}, {177.0, 15711553}, {178.0, 15843139}, {179.0, 15974213}, {180.0, 15974215}, {181.0, 15974217}, {182.0, 15974219}, {183.0, 15975755}, {184.0, 15976271}, {185.0, 15976785}, {186.0, 15977299}, {187.0, 15977301}, {188.0, 15977815}, {189.0, 15978327}, {190.0, 15978331}, {191.0, 16109917}, {192.0, 16241503}, {193.0, 16241505}, {194.0, 16242019}, {195.0, 16242535}, {196.0, 16242537}, {197.0, 16242539}, {198.0, 16243563}, {199.0, 16243567}, {200.0, 16244081}, {201.0, 16244595}, {202.0, 16244599}, {203.0, 16244601}, {204.0, 16244603}, {205.0, 16245627}, {206.0, 16245631}, {207.0, 16245633}, {208.0, 16246147}, {209.0, 16246663}, {210.0, 16377735}, {211.0, 16508811}, {212.0, 16508815}, {213.0, 16509839}, {214.0, 16509843}, {215.0, 16509845}, {216.0, 16509847}, {217.0, 16510361}, {218.0, 16510875}, {219.0, 16510879}, {220.0, 16510881}, {221.0, 16510883}, {222.0, 16511399}, {223.0, 16511911}, {224.0, 16511915}, {225.0, 16511917}, {226.0, 16511919}, {227.0, 16511923}, {228.0, 16512437}, {229.0, 16512951}, {230.0, 16512955}, {231.0, 16512957}, {232.0, 16512959}, {233.0, 16512961}, {234.0, 16512963}, {235.0, 16512967}, {236.0, 16513481}, {237.0, 16513995}, {238.0, 16513999}, {239.0, 16514001}, {240.0, 16514003}, {241.0, 16514005}, {242.0, 16514007}, {243.0, 16514011}, {244.0, 16514013}, {245.0, 16514015}, {246.0, 16514019}, {247.0, 16514021}, {248.0, 16514023}, {249.0, 16514027}, {250.0, 16514029}, {251.0, 16514031}, {252.0, 16514035}, {253.0, 16514037}, {254.0, 16514039}, {255.0, 16514043}] ("Z Scale.Marker Values[]")] -> w638
                  tunnel: w642 -> [w648 w650 w652 w654 w656 w658 w660 w662 w664 w666 w668 w671]
                  tunnel: [w648 w650 w652 w654 w656 w658 w660 w662 w664 w666 w668 w671] -> w640
                  frame "Fire", Default {
                    # "Fire"
                  }
                  frame "Gray" {
                    # "Grayscale"
                  }
                  frame "Red" {
                    # "Red"
                  }
                  frame "Green" {
                    # "Green"
                  }
                  frame "Blue" {
                    # "Blue"
                  }
                  frame "Cyan" {
                    # "Cyan"
                  }
                  frame "Magenta" {
                    # "Magenta"
                  }
                  frame "Yellow" {
                    # "Yellow"
                  }
                  frame "Red-White" {
                    # "Red-White"
                  }
                  frame "Green-White" {
                    # "Green-White"
                  }
                  frame "Blue-White" {
                    # "Blue-White"
                  }
                  frame "Glow" {
                  }
                }
                n320 = property on="Apply Color" class="Bool (strict)"(error in=w636, "Value"=FALSE) -> ()  [unwired: 1 in, 2 out]
                n321 = property class="IntGraph (strict)"(reference=w639, "ZScale.MarkerVals[]"=w638, "ZScale.High Color"=u32 255, "ZScale.Maximum"=w640) -> ()  [unwired: 1 in, 2 out]
              }
              frame "Show Cursor", Default {
                w676 = 2.0 ("y")
                n322 = Index Array(array=w672, index=0) -> (element=w684:refnum<vi>)
                n323 = property class="IntGraph (strict)"(reference=w684) -> ("Value"=w683:sgl[][])  [unwired: 1 in, 2 out]
                n324 = Array Size(array=w683) -> (size(s)=w682:i32[])
                n325 = To Double Precision Float(number=w682) -> (double precision float=w679:dbl[])
                n326 = Index Array(array=w679, index #1=0 ("index"), index #2=1 ("index")) -> (element #1=w678:dbl, element #2=w677:dbl)
                n327 = Divide(x=w678, y=w676) -> (x/y=w675:dbl)
                n328 = Divide(x=w677, y=w676) -> (x/y=w674:dbl)
                n329 = for {
                  tunnel: w672 -> [w686] mode=indexing
                  tunnel: w675 -> [w688]
                  tunnel: w674 -> [w687]
                  tunnel: w673 -> [w689]
                  n330 = property class="IntGraph (strict)"(reference=w686, "Cursor.Visible"=w689, "Cursor.Cursor X"=w688, "Cursor.Cursor Y"=w687) -> ()  [unwired: 1 in, 2 out]
                }
              }
              frame "Auto Scale" {
                n331 = Select(t=u8 2 ("Z Scale.Scale Fit"), s=w693, f=u8 0) -> (s? t:f=w690:u8)
                n332 = for {
                  tunnel: w694 -> [w696] mode=indexing
                  tunnel: w690 -> [w695]
                  n333 = property class="IntGraph (strict)"(reference=w696, "ZScale.ScaleFit"=w695) -> ()  [unwired: 1 in, 2 out]
                }
              }
              frame "Pan Tool", "Reset Zoom", "Zoom In", "Zoom Out" {
                n334 = case shown="\"Reset Zoom\"" w704 {
                  tunnel: [0 ("Palette:Active Tool") 6 ("Palette:Active Tool") 7 ("Palette:Active Tool") 1 ("Palette:Active Tool") 0 ("Palette:Active Tool")] -> w698
                  tunnel: w697 -> [_ _ _ _ w716]
                  frame Default {
                  }
                  frame "Zoom In" {
                  }
                  frame "Zoom Out" {
                  }
                  frame "Pan Tool" {
                  }
                  frame "Reset Zoom" {
                    n335 = property on="Reset Zoom" class="Bool (strict)"("Value"=FALSE) -> ()  [unwired: 2 in, 2 out]
                    n336 = for {
                      tunnel: w716 -> [w721] mode=indexing
                      tunnel: 5 ("Palette:Active Tool") -> [w720]
                      n337 = property class="IntGraph (strict)"(reference=w721, "ActPaletteTool"=w720) -> ()  [unwired: 1 in, 2 out]
                    }
                  }
                }
                n338 = control-ref of="Zoom In"() -> (w700:refnum<vi>)
                n339 = control-ref of="Zoom Out"() -> (w702:refnum<vi>)
                n340 = control-ref of="Pan Tool"() -> (w701:refnum<vi>)
                n341 = Build Array(w700, w702, w701) -> (w703:refnum<vi>[])
                n342 = for {
                  tunnel: w703 -> [w709] mode=indexing
                  tunnel: w699 -> [w707]
                  n343 = property class="Bool (strict)"(reference=w709) -> (reference out=w708:refnum<vi>, "Label.Text"=w706:string)  [unwired: 1 in, 1 out]
                  n344 = Equal?(x=w706, y=w707) -> (x = y?=w705:bool)
                  n345 = property class="Bool (strict)"(reference=w708, "Value"=w705) -> ()  [unwired: 1 in, 2 out]
                }
                n346 = for {
                  tunnel: w697 -> [w711] mode=indexing
                  tunnel: w698 -> [w710]
                  n347 = property class="IntGraph (strict)"(reference=w711, "ActPaletteTool"=w710) -> ()  [unwired: 1 in, 2 out]
                }
              }
              frame "Load File" {
                w731 = u16 1 items=["Get Image", "Load and Read File"] ("Action")
                n348 = control-ref of="This VI"() -> (w733:refnum<vi>)
                n349 = property on="Load File" class="Bool (strict)"("Value"=FALSE) -> ()  [unwired: 2 in, 2 out]
                n350 = call "GetDisplayClick.vi"("Display REFs In"=w734, "Calling VI REF"=w733) -> ("Display Index"=w722:i32)  [unwired: 13 in]
                n351 = call "OpenDBL.vi"("Action"=w731) -> ("Image"=w730:sgl[], "Dimensions (Z, Y, X, t)"=w729:i32[])  [unwired: 12 in, 1 out]
                n352 = Index Array(array=w729, index #1=1 ("index"), index #2=2 ("index")) -> (element #1=w726:i32, element #2=w725:i32)
                n353 = Reverse 1D Array(array=w730) -> (reversed array=w724:sgl[])
                n354 = Reshape Array(w724, w726, w725) -> (w723:sgl[][])
                n355 = Index Array(array=w734, index=w722) -> (element=w732:refnum<vi>)
                n356 = property class="IntGraph (strict)"(reference=w732, "Value"=w723) -> ()  [unwired: 1 in, 2 out]
              }
              frame "Fit Tool" {
                n357 = disable-structure shown="Disabled" {
                  frame Disabled {
                    n358 = vi-ref "QuickProfile_V4.vi"() -> (w738:refnum<vi>)
                    n359 = call "Image Aquisition Param Ctrl_AE.vi"("Action"=enum16{"READ", "WRITE"}."READ") -> ()  [unwired: 10 in, 1 out]
                    n360 = property class="VI Interface Type 0"(reference=w738) -> ("Path"=w741:path)  [unwired: 1 in, 2 out]
                    n361 = Unbundle By Name() -> ("Pixel Size (nm)"=w737:dbl[])  [unwired: 1 in]
                    n362 = Index Array(array=w737, index=0) -> (element=w744:dbl)
                    n363 = Open VI Reference(type specifier VI Refnum (for type only)=w738, vi path=w741, options=128) -> (vi reference=w739:refnum<vi>)  [unwired: 3 in, 1 out]
                    n364 = call-by-ref "Start Asynchronous Call"(reference=w739, "Pixel Size (nm)"=w744) -> (reference out=w742:refnum<vi>)  [unwired: 16 in, 1 out]
                    n365 = Close Reference(reference=w742) -> ()  [unwired: 1 in, 1 out]
                  }
                  frame Enabled {
                  }
                }
              }
              frame "Smooth Tool" {
                n366 = vi-ref "SmoothTool.vi"() -> (w749:refnum<vi>)
                n367 = property on="Smooth Tool" class="Bool (strict)"("Value"=FALSE) -> ()  [unwired: 2 in, 2 out]
                n368 = property class="VI Interface Type 1"(reference=w749) -> ("Path"=w751:path)  [unwired: 1 in, 2 out]
                n369 = control-ref of="This VI"() -> (w747:refnum<vi>)
                n370 = Open VI Reference(type specifier VI Refnum (for type only)=w749, vi path=w751, options=128) -> (vi reference=w750:refnum<vi>)  [unwired: 3 in, 1 out]
                n371 = call-by-ref "Start Asynchronous Call"(reference=w750, "Calling VI REF"=w747, "Display REFs In"=w746) -> (reference out=w748:refnum<vi>)  [unwired: 11 in, 1 out]
                n372 = Close Reference(reference=w748) -> ()  [unwired: 1 in, 1 out]
              }
              frame "Merge Tool" {
                n373 = vi-ref "MergeTool - Cambridge.vi"() -> (w757:refnum<vi>)
                n374 = property class="VI Interface Type 2"(reference=w757) -> ("Path"=w759:path)  [unwired: 1 in, 2 out]
                n375 = property on="Merge Tool" class="Bool (strict)"("Value"=FALSE) -> ()  [unwired: 2 in, 2 out]
                n376 = control-ref of="This VI"() -> (w755:refnum<vi>)
                n377 = Open VI Reference(type specifier VI Refnum (for type only)=w757, vi path=w759, options=128) -> (vi reference=w758:refnum<vi>)  [unwired: 3 in, 1 out]
                n378 = call-by-ref "Start Asynchronous Call"(reference=w758, "VI Reference"=w755, "Display References"=w754) -> (reference out=w756:refnum<vi>)  [unwired: 11 in, 1 out]
                n379 = Close Reference(reference=w756) -> ()  [unwired: 1 in, 1 out]
              }
            }
          }
        }
      }
      event "Channel 1", "Channel 2", "Channel 3", "Channel 4", "Channel 5", "Channel 6": Mouse Down; "Channel 1", "Channel 2", "Channel 3", "Channel 4", "Channel 5", "Channel 6": Mouse Up {
        n380 = event-data() -> ("Type"=w766:T23, "CtlRef"=w763:refnum<vi>)  [unwired: 1 in, 5 out]
        n381 = Equal?(x=w766, y=lveventtype."Mouse Down" ("Type")) -> (x = y?=w764:bool)
        n382 = call "Graph Ref AE.vi"("Action"=enum16{"READ", "WRITE"}."READ") -> ("Graph Ref Out"=w761:refnum<vi>[])  [unwired: 10 in]
        n383 = case shown="True" w764 {
          tunnel: w763 -> [w769 w787]
          tunnel: w761 -> [w768 w786]
          frame False {
            n384 = property class="IntGraph (strict)"(reference=w769) -> (reference out=w773:refnum<vi>, "ActPaletteTool"=w770:i32)  [unwired: 1 in, 1 out]
            n385 = Not Equal?(x=w770, y=0) -> (x != y?=w772:bool)
            n386 = case shown="False" w772 {
              tunnel: w773 -> [w776 w782]
              tunnel: w768 -> [w775 w779]
              frame False {
                n387 = property class="IntGraph (strict)"(reference=w776) -> ("Cursor.Cursor Position"=w774:T33)  [unwired: 1 in, 2 out]
                n388 = for {
                  tunnel: w775 -> [w777] mode=indexing
                  tunnel: w774 -> [w778]
                  n389 = property class="IntGraph (strict)"(reference=w777, "Cursor.Cursor Position"=w778) -> ()  [unwired: 1 in, 2 out]
                }
              }
              frame True {
                n390 = property class="IntGraph (strict)"(reference=w782) -> ("XScale.Range"=w781:T34, "YScale.Range"=w780:T34)  [unwired: 1 in, 2 out]
                n391 = for {
                  tunnel: w781 -> [w785]
                  tunnel: w780 -> [w784]
                  tunnel: w779 -> [w783] mode=indexing
                  n392 = property class="IntGraph (strict)"(reference=w783, "XScale.Range"=w785, "YScale.Range"=w784) -> ()  [unwired: 1 in, 2 out]
                }
              }
            }
          }
          frame True {
            n393 = for {
              tunnel: w786 -> [w792] mode=indexing
              tunnel: w787 -> [w793]
              n394 = Equal?(x=w792, y=w793) -> (x = y?=w791:bool)
              n395 = Select(t=T24 {"Left"=2431, "Top"=-324} ("Z Scale.Position"), s=w791, f=T24 {"Left"=0, "Top"=0}) -> (s? t:f=w788:T24)
              n396 = property class="IntGraph (strict)"(reference=w792, "ZScale.Visible"=w791, "ZScale.Position"=w788) -> ()  [unwired: 1 in, 2 out]
            }
          }
        }
      }
      event "Load Positions": Value Change {
        n397 = event-data() -> ()  [unwired: 1 in, 6 out]
        n398 = call "Load Stage Positions.vi"() -> ("appended array"=w806:bool[])  [unwired: 1 in]
        n399 = control-ref of="Abort AllStage"() -> (w804:refnum<vi>)
        n400 = Build Array("P841", "M686", "M686", "P612") -> (w805:string[])
        n401 = TDMS Open(10:T25."open (read-only)" ("operation (0:open)"), 11:path "C:/Users/ED STED/Documents/Test Control Software/Host VIs/Stages/Stage Positions/Stage Positions in Last Experiment.tdms" ("file path")) -> (3:w800:refnum<k34>)  [unwired: 5 in, 1 out]
        n402 = TDMS Read(0:w800, 5:"Stage Positions" ("group name in (Untitled)")) -> (4:w799:refnum<k34>, 10:w797:waveform(dbl)[])  [unwired: 6 in, 4 out]
        n403 = Index Array(array=w797, index=0) -> (element=w795:waveform(dbl))
        n404 = TDMS Close(11:w799) -> ()  [unwired: 1 in, 2 out]
        n405 = Unbundle By Name(w795) -> ("Y"=w794:dbl[])
        n406 = for {
          N -> [w812]
          tunnel: w806 -> [w815] mode=indexing
          tunnel: w805 -> [w814] mode=indexing
          tunnel: w804 -> [w813]
          tunnel: w794 -> [w811] mode=indexing
          n407 = case shown="True" w815 {
            tunnel: w814 -> [_ w818]
            tunnel: w813 -> [_ w819]
            tunnel: w812 -> [_ w817]
            tunnel: w811 -> [_ w816]
            frame False {
            }
            frame True {
              n408 = case shown="\"M686\"" w818 {
                tunnel: w819 -> [w823 w847 w875]
                tunnel: w818 -> [w824 w848 w876]
                tunnel: w817 -> [_ w844 w872]
                tunnel: w816 -> [w821 w843 w871]
                frame "P612", Default {
                  n409 = flat-sequence {
                    tunnel: w824 -> [w835]
                    tunnel: w823 -> [w836]
                    tunnel: [w836] -> w822
                    tunnel: w821 -> [w825]
                    tunnel: [w835] -> w820
                    tunnel: w822 -> [w841]
                    tunnel: w820 -> [w838]
                    frame #0 {
                      n410 = Divide(x=w825, y=10.0) -> (x/y=w828:dbl)
                      n411 = call "Volts to I16.vi"("Voltage (V)"=w828) -> ("I16"=w829:i16)  [unwired: 13 in, 1 out]
                      n412 = call "Manual Controls Action Engine.vi"("Action"=enum16{"Read", "Write"}."Read") -> ("Manual Controls Out"=w830:T17)  [unwired: 14 in]
                      n413 = Bundle By Name(cluster=w830, "Z Axis Voltage (I16)"=w829) -> (w833:T17)
                      n414 = call "Manual Controls Action Engine.vi"("Action"=enum16{"Read", "Write"}."Write", "Manual Controls In"=w833) -> ()  [unwired: 13 in, 1 out]
                      n415 = call "FPGA-7842R-Control V1.vi"("Action"=FPGA-7842R-Reference."Stage Control", "Manual Controls"=w833, "Initialize"=TRUE) -> ()  [unwired: 11 in, 2 out]
                    }
                    frame #1 {
                      n416 = call "AE_AllStages_Action V2.vi"("Abort"=w841, "Axis"=bool[] [TRUE, TRUE, TRUE], "Stage ID"=w838, "Action"=StageStates."POSITION") -> ("Position Out"=w840:dbl[])  [unwired: 5 in, 2 out]
                      n417 = Index Array(array=w840, index=2) -> ()  [unwired: 1 out]
                    }
                  }
                }
                frame "M686" {
                  n418 = flat-sequence {
                    tunnel: w848 -> [w860]
                    tunnel: w847 -> [w855]
                    tunnel: [w855] -> w846
                    tunnel: [w853] -> w845
                    tunnel: w844 -> [w852]
                    tunnel: w843 -> [w849]
                    tunnel: w846 -> [w869]
                    tunnel: w845 -> [w867]
                    frame #0 {
                      w853 = bool[] [TRUE, TRUE] ("Axis")
                      n419 = call "AE_AllStages_Action V2.vi"("Abort"=w855, "Axis"=w853, "Stage ID"=w860, "Action"=StageStates."POSITION") -> ("Position Out"=w859:dbl[])  [unwired: 5 in, 2 out]
                      n420 = Subtract(x=w852, y=1) -> (x-y=w850:i32)
                      n421 = Replace Array Subset(array=w859, new element=w849, index=w850) -> (w858:dbl[])
                      n422 = call "AE_AllStages_Action V2.vi"("Velocity"=1.0, "Abort"=w855, "Positions"=w858, "Axis"=w853, "Stage ID"="M686", "Action"=StageStates."MOVE") -> ()  [unwired: 3 in, 3 out]
                    }
                    frame #1 {
                      n423 = call "AE_AllStages_Action V2.vi"("Abort"=w869, "Axis"=w867, "Stage ID"="M686", "Action"=StageStates."POSITION") -> ("Position Out"=w866:dbl[])  [unwired: 5 in, 2 out]
                      n424 = Index Array(array=w866, index #1=0 ("index"), index #2=1 ("index")) -> (element #1=w864:dbl, element #2=w862:dbl)
                      n425 = property on="X" class="DigNum (strict)"("Value"=w864) -> ()  [unwired: 2 in, 2 out]
                      n426 = property on="Y" class="DigNum (strict)"("Value"=w862) -> ()  [unwired: 2 in, 2 out]
                    }
                  }
                }
                frame "P841" {
                  n427 = flat-sequence {
                    tunnel: w876 -> [_]
                    tunnel: w875 -> [w881]
                    tunnel: [w881] -> w874
                    tunnel: [w879] -> w873
                    tunnel: w872 -> [_]
                    tunnel: w871 -> [w877]
                    tunnel: w874 -> [w889]
                    tunnel: w873 -> [w887]
                    frame #0 {
                      w879 = bool[] [TRUE] ("Axis")
                      n428 = Build Array(w877) -> (w878:dbl[])
                      n429 = call "AE_AllStages_Action V2.vi"("Velocity"=1.0, "Abort"=w881, "Positions"=w878, "Axis"=w879, "Stage ID"="P841", "Action"=StageStates."MOVE") -> ()  [unwired: 3 in, 3 out]
                    }
                    frame #1 {
                      n430 = call "AE_AllStages_Action V2.vi"("Abort"=w889, "Axis"=w887, "Stage ID"="P841", "Action"=StageStates."POSITION") -> ("Position Out"=w886:dbl[])  [unwired: 5 in, 2 out]
                      n431 = Index Array(array=w886, index #1=0 ("index")) -> (element #1=w884:dbl)  [unwired: 1 in, 1 out]
                      n432 = property on="Position (µm)" class="DigNum (strict)"("Value"=w884) -> ()  [unwired: 2 in, 2 out]
                    }
                  }
                }
              }
            }
          }
        }
      }
      event "Exit": Value Change {
        n433 = event-data() -> ("CtlRef"=w902:refnum<vi>, "NewVal"=w904:bool)  [unwired: 1 in, 1 out]
        n434 = disable-structure shown="Disabled" {
          frame Disabled {
            n435 = Two Button Dialog(message="Record the positions of piezo stages?", 1:"No" ("F button name (\"Cancel\")"), 2:"Yes" ("T button name (\"OK\")")) -> (T button?=w905:bool)
            n436 = case shown="True" w905 {
              frame False {
              }
              frame True {
                n437 = Build Array("P612" ("Stage ID"), "M686" ("Stage ID"), "P841" ("Stage ID")) -> (w913:string[])
                n438 = for {
                  tunnel: w913 -> [w920] mode=indexing
                  tunnel: [w919] -> w909 mode=concatenating
                  n439 = call "Stage_position_ae.vi"("StageID"=w920, "Enum"=enum16{"WRITE", "READ"}."READ") -> ("Position Out"=w919:dbl[])  [unwired: 8 in, 1 out]
                }
                n440 = TDMS Open(10:T25."create or replace" ("operation (0:open)"), 11:path "C:/Users/ED STED/Documents/Test Control Software/Host VIs/Stages/Stage Positions/Stage Positions in Last Experiment.tdms" ("file path")) -> (3:w915:refnum<k34>)  [unwired: 5 in, 1 out]
                n441 = TDMS Write(0:w915, 5:"Stage Positions" ("group name in (Untitled)"), 9:w909) -> (4:w916:refnum<k34>)  [unwired: 3 in, 3 out]
                n442 = TDMS Close(11:w916) -> ()  [unwired: 1 in, 2 out]
              }
            }
          }
          frame Enabled {
          }
        }
        n443 = Release Notifier(notifier=w897, force destroy? (F)=TRUE) -> ()  [unwired: 1 in, 3 out]
        n444 = property class="Bool"(reference=w902) -> ("Label.Text"=w901:string)  [unwired: 1 in, 2 out]
        n445 = call "SLM AE.vi"("Action"=enum16{"READ", "WRITE"}."READ") -> ("SLM Ref Out"=w895:refnum<vi>)  [unwired: 10 in]
        n446 = call "DM_Ref_AE.vi"("Action"=enum16{"READ", "WRITE"}."READ") -> ("DM Ref Out"=w893:refnum<vi>)  [unwired: 10 in]
        n447 = call "GateDelay AE.vi"("Action"=enum16{"READ", "WRITE"}."READ") -> ("Gate Delay Ref Out"=w894:refnum<vi>)  [unwired: 10 in]
        n448 = Enqueue Element(queue=w903, element=w901) -> ()  [unwired: 2 in, 3 out]
        n449 = Build Array(w895, w893, w894) -> (w892:refnum<vi>[])
        n450 = for {
          tunnel: w892 -> [w926] mode=indexing
          n451 = Not A Number/Path/Refnum?(number/path/refnum=w926) -> (NaN/Path/Refnum?=w925:bool)
          n452 = case shown="False" w925 {
            tunnel: w926 -> [w927 _]
            frame False {
              n453 = To Variant(anything=TRUE) -> (Variant=w928:variant)
              n454 = invoke class="VI" method="Ctrl Val.Set"(reference=w927, "Control Name"="Exit", "Value"=w928) -> (reference out=w931:refnum<vi>)  [unwired: 2 in, 4 out]
              n455 = Close Reference(reference=w931) -> ()  [unwired: 1 in, 1 out]
            }
            frame True {
            }
          }
        }
        n456 = property on="Stages" class="Clust (strict)"() -> ("Controls[]"=w891:refnum<vi>[])  [unwired: 2 in, 2 out]
        n457 = for {
          tunnel: w891 -> [w924] mode=indexing
          n458 = property class="Ctl"(reference=w924) -> ("Label.Text"=w923:string)  [unwired: 1 in, 2 out]
          n459 = call "All_Stages_Aloha.vi"("Aloha"=FALSE, "Stage ID"=w923) -> ()  [unwired: 9 in, 1 out]
        }
      }
    }
  }
  n460 = disable-structure shown="Disabled" {
    frame Disabled {
    }
    frame Enabled {
    }
  }
  n461 = call "Manual Controls Action Engine.vi"("Action"=enum16{"Read", "Write"}."Write", "Manual Controls In"=w27) -> ("Manual Controls Out"=w29:T17)  [unwired: 13 in]
  n462 = call "FPGA-7842R-Control V1.vi"("Action"=FPGA-7842R-Reference."Initialize", "Manual Controls"=w29, "Initialize"=FALSE) -> ("Initalized"=w11:bool)  [unwired: 11 in, 1 out]
  n463 = while {
    shift-right: [w941] -> _
    shift-left: "Idle" -> [w942]
    tunnel: w18 -> [w938]
    shift-right: [w936] -> _
    shift-left: w11 -> [w937]
    stop <- w940 stop-if-true
    n464 = call "Image Aquisition Param Ctrl_AE.vi"("Action"=enum16{"READ", "WRITE"}."READ") -> ("Image Acquisition Parameters Out"=w935:T15)  [unwired: 10 in]
    n465 = call "Detectors Crl_AE.vi"("Action"=enum16{"READ", "WRITE"}."READ") -> ("Detectors Parameters Out"=w933:T13)  [unwired: 10 in]
    n466 = case shown="\"Arange Displays\"" w942 {
      selector: w942 -> [_ _ _ w974 _ _ _ _ _ _]
      tunnel: ["Exit" w951 "Idle" ("name (unnamed)") "Arange Displays" ("name (unnamed)") "Start FPGA Acquisition" ("name (unnamed)") "Display" ("name (unnamed)") "Close Images" ("name (unnamed)") "Idle" "Stop Waveforms" ("name (unnamed)") "Start Waveforms" ("name (unnamed)")] -> w941
      tunnel: [TRUE w953 w960 w982 w998 w1019 w1060 w1093 w1098 w1104] -> w940
      tunnel: FALSE -> [_ w953 w960 w982 w998 w1019 w1060 w1093 w1098 w1104]
      tunnel: w938 -> [_ w952 _ _ _ _ _ _ _ _]
      tunnel: w937 -> [w947 w950 w961 w980 w995 w1017 w1058 w1091 w1099 w1105]
      tunnel: [w946 w950 w961 w980 w995 w1013 w1058 w1090 w1099 w1105] -> w936
      tunnel: w935 -> [_ _ _ w973 _ w1012 _ _ _ w1102]
      tunnel: w933 -> [_ _ _ w972 _ _ _ _ _ w1100]
      frame "Exit" {
        n467 = call "Graph Ref AE.vi"("Action"=enum16{"READ", "WRITE"}."READ") -> ("Graph Ref Out"=w944:refnum<vi>[])  [unwired: 10 in]
        n468 = call "FPGA-7842R-Control V1.vi"("Action"=FPGA-7842R-Reference."Close FPGA", "Initialize"=w947) -> ("Initalized"=w946:bool)  [unwired: 12 in, 1 out]
        n469 = Close Reference(reference=w944) -> ()  [unwired: 1 in, 1 out]
      }
      frame "Idle", Default {
        n470 = Dequeue Element(queue=w952, timeout in ms (-1)=-1) -> (element=w951:string)  [unwired: 1 in, 3 out]
      }
      frame "Close Images" {
        w956 = u16 0 items=["Read", "Write"] ("Mode")
        w957 = u16 0 items=["Write", "Read"] ("Mode")
        n471 = call "File Action V1.vi"("Mode"=w956) -> ("Files Open"=w955:bool)  [unwired: 12 in, 2 out]
        n472 = call "Image_Actions_V1.vi"("Mode"=w957, "Action"="Trash Images") -> ()  [unwired: 12 in, 2 out]
        n473 = case shown="True" w955 {
          frame False {
          }
          frame True {
            w963 = u16 1 items=["Read", "Write"] ("Mode")
            n474 = call "File Action V1.vi"("Action"="Close Files", "Mode"=w963) -> ()  [unwired: 11 in, 3 out]
          }
        }
      }
      frame "Capture", "Live" {
        w978 = u16 0 items=["Write", "Read"] ("Mode")
        n475 = Cluster To Array(cluster=w972) -> (array=w970:bool[])
        n476 = Index Array(array=w970, index=4) -> (element=w967:bool)
        n477 = Boolean To (0,1)(Boolean=w970) -> (0, 1=w971:i16[])
        n478 = Add Array Elements(numeric array=w971) -> (sum=w968:i16)
        n479 = To Long Integer(number=w968) -> (32bit integer=w965:i32)
        n480 = Unbundle By Name(w973) -> ("Image Format"=w975:u16)
        n481 = Select(t=1, s=w967, f=w965) -> (s? t:f=w964:i32)
        n482 = case shown="\"Capture\"" w974 {
          tunnel: w973 -> [_ w984]
          tunnel: w964 -> [_ w983]
          frame Default {
          }
          frame "Capture" {
            w987 = u16 1 items=["Read", "Write"] ("Mode")
            n483 = call "File Action V1.vi"("Action"="Open Files", "Mode"=w987, "Image Acquisition Parameters"=w984, "File Path IN"="Save File Path", "Number of Channels"=w983) -> ("File Path OUT"=w985:path)  [unwired: 8 in, 2 out]
            n484 = local write "Save File Path"(w985) -> ()
          }
        }
        n485 = To Long Integer(number=w975) -> (32bit integer=w977:i32)
        n486 = Bundle(w977, w977) -> (w976:cluster{i32, i32})  [unwired: 1 in]
        n487 = call "Image_Actions_V1.vi"("Image Size (Pixels)"=w976, "Mode"=w978, "Number of Channels"=w964, "Action"="Create Images") -> ()  [unwired: 10 in, 2 out]
      }
      frame "Arange Displays" {
        w993 = u16 1 items=["Write", "Read"] ("Mode")
        w996 = u16 1 items=["Read", "Write"] ("Action")
        n488 = call "Graph Ref AE.vi"("Action"=enum16{"READ", "WRITE"}."READ") -> ("Graph Ref Out"=w989:refnum<vi>[])  [unwired: 10 in]
        n489 = call "Image_Actions_V1.vi"("Mode"=w993) -> ("Image REFs OUT"=w994:T35[])  [unwired: 13 in, 1 out]
        n490 = Array Size(array=w994) -> (size(s)=w992:i32)
        n491 = call "Arange_Displays_V2.vi"("Display References"=w989, "Action"=w996, "Number of Channels"=w992, "Aspect Ratio (h/w)"=1.0) -> ("Number of Channels OUT"=w990:i32)  [unwired: 11 in]
        n492 = for {
          N: w990 -> [_]
          tunnel: w989 -> [w1000] mode=indexing
          tunnel: [w1003] -> _ mode=indexing
          i -> [w1001]
          n493 = property class="IntGraph (strict)"(reference=w1000) -> ("Label.Text"=w1005:string)  [unwired: 1 in, 2 out]
          n494 = Equal To 0?(x=w1001) -> (x = 0?=w1002:bool)
          n495 = case shown="True" w1002 {
            tunnel: w1000 -> [_ w1006]
            frame False {
            }
            frame True {
              n496 = property class="IntGraph (strict)"(reference=w1006, "ZScale.Visible"=TRUE ("Z Scale.Visible"), "ZScale.Position"=T24 {"Left"=2431, "Top"=-324} ("Z Scale.Position")) -> ()  [unwired: 1 in, 2 out]
            }
          }
          n497 = To Unsigned Word Integer(number=w1001) -> (unsigned 16bit integer=w1004:u16)
          n498 = Bundle("Label.Text"=w1005, w1004) -> (w1003:cluster{"Label.Text":string, u16})  [unwired: 1 in]
        }
      }
      frame "Start Waveforms" {
        n499 = call "Initialize Waveforms V4.vi"("Image Acquisition Parameters"=w1012) -> ("Waveform Data to FPGA"=w1018:T36)  [unwired: 14 in]
        n500 = Unbundle By Name(w1012) -> ("Scan Type"=w1011:enum16{"Sample Scanning", "Beam Scanning"})
        n501 = call "FPGA-7842R-Control V1.vi"("Waveform Data"=w1018, "Action"=FPGA-7842R-Reference."Start Waveforms", "Image Acquisition Parameters"=w1012, "Initialize"=w1017) -> ("Initalized"=w1014:bool)  [unwired: 10 in, 1 out]
        n502 = Equal?(x=w1011, y=enum16{"Sample Scanning", "Beam Scanning"}."Sample Scanning" ("Scan Type")) -> (x = y?=w1009:bool)
        n503 = case shown="False" w1009 {
          tunnel: w1014 -> [w1020 w1025]
          tunnel: [w1020 w1024] -> w1013
          frame False {
          }
          frame True {
            n504 = call "Scan Parameters Action Engine.vi"("Action"=enum16{"Read", "Write"}."Read") -> ("Scan Parameters OUT"=w1022:T16)  [unwired: 14 in]
            n505 = Unbundle By Name(w1022) -> ("Unused_Axis_I16"=w1021:i16)
            n506 = call "FPGA-7842R-Control V1.vi"("Action"=FPGA-7842R-Reference."Unused Axis I16", "Initialize"=w1025, "Unused Axis Offset (I16)"=w1021) -> ("Initalized"=w1024:bool)  [unwired: 11 in, 1 out]
          }
        }
      }
      frame "Display" {
        w1053 = u16 1 items=["Write", "Read"] ("Mode")
        n507 = call "Image_Actions_V1.vi"("Mode"=w1053) -> ("Image REFs OUT"=w1055:T35[])  [unwired: 13 in, 1 out]
        n508 = Array Size(array=w1055) -> (size(s)=w1051:i32)
        n509 = Decrement(x=w1051) -> (x-1=w1050:i32)
        n510 = for {
          N: 6 -> [_]
          tunnel: w1050 -> [w1088]
          tunnel: [w1086] -> w1054 mode=indexing
          i -> [w1087]
          n511 = Greater Or Equal?(x=w1088, y=w1087) -> (x >= y?=w1086:bool)
        }
        n512 = Obtain Notifier(name (unnamed)="Running", notification data type=FALSE) -> (notifier out=w1027:refnum<notifier>)  [unwired: 2 in, 2 out]
        n513 = Index Array(array=w1054, index #1=1 ("index"), index #2=2 ("index"), index #3=3 ("index"), index #4=4 ("index"), index #5=5 ("index")) -> (element #1=w1039:bool, element #2=w1038:bool, element #3=w1037:bool, element #4=w1036:bool, element #5=w1035:bool)
        n514 = Index Array(array=w1055, index #1=0 ("index"), index #2=1 ("index"), index #3=2 ("index"), index #4=3 ("index"), index #5=4 ("index"), index #6=5 ("index")) -> (element #1=w1034:T35, element #2=w1033:T35, element #3=w1032:T35, element #4=w1031:T35, element #5=w1030:T35, element #6=w1029:T35)
        n515 = while {
          tunnel: w1039 -> [w1075]
          tunnel: w1038 -> [w1074]
          tunnel: w1037 -> [w1070]
          tunnel: w1036 -> [w1067]
          tunnel: w1035 -> [w1066]
          tunnel: w1034 -> [w1073]
          tunnel: w1033 -> [w1072]
          tunnel: w1032 -> [w1071]
          tunnel: w1031 -> [w1069]
          tunnel: w1030 -> [w1065]
          tunnel: w1029 -> [w1068]
          tunnel: w1027 -> [w1062]
          stop <- w1063 stop-if-true
          n516 = Get Notifier Status(notifier=w1062) -> (current notification=w1063:bool)  [unwired: 1 in, 4 out]
          n517 = case shown="True" w1075 {
            tunnel: w1072 -> [_ w1085]
            frame False {
            }
            frame True {
              n518 = call "IMAQ ImageToArray"("Image"=w1085) -> ("Image Pixels (Float)"=→"Channel 2":sgl[][])  [unwired: 3 in, 4 out]
            }
          }
          n519 = case shown="True" w1074 {
            tunnel: w1071 -> [_ w1083]
            frame False {
            }
            frame True {
              n520 = call "IMAQ ImageToArray"("Image"=w1083) -> ("Image Pixels (Float)"=→"Channel 3":sgl[][])  [unwired: 3 in, 4 out]
            }
          }
          n521 = call "IMAQ ImageToArray"("Image"=w1073) -> ("Image Pixels (Float)"=→"Channel 1":sgl[][])  [unwired: 3 in, 4 out]
          n522 = case shown="True" w1070 {
            tunnel: w1069 -> [_ w1081]
            frame False {
            }
            frame True {
              n523 = call "IMAQ ImageToArray"("Image"=w1081) -> ("Image Pixels (Float)"=→"Channel 4":sgl[][])  [unwired: 3 in, 4 out]
            }
          }
          n524 = case shown="False" w1067 {
            tunnel: w1065 -> [_ w1079]
            frame False {
            }
            frame True {
              n525 = call "IMAQ ImageToArray"("Image"=w1079) -> ("Image Pixels (Float)"=→"Channel 5":sgl[][])  [unwired: 3 in, 4 out]
            }
          }
          n526 = case shown="True" w1066 {
            tunnel: w1068 -> [_ w1077]
            frame False {
            }
            frame True {
              n527 = call "IMAQ ImageToArray"("Image"=w1077) -> ("Image Pixels (Float)"=→"Channel 6":sgl[][])  [unwired: 3 in, 4 out]
            }
          }
          n528 = Wait (ms)(milliseconds to wait=u32 100) -> ()  [unwired: 1 out]
        }
      }
      frame "Stop Waveforms" {
        n529 = call "FPGA-7842R-Control V1.vi"("Action"=FPGA-7842R-Reference."Stop Waveforms", "Initialize"=w1091) -> ("Initalized"=w1090:bool)  [unwired: 12 in, 1 out]
      }
      frame "Stop Acquisition" {
        n530 = call "FPGA-7842R-Control V1.vi"("Action"=FPGA-7842R-Reference."Laser Control", "Laser Controls"=T14 {"STED Power (V)"=0.0, "STED"=FALSE, "640 nm"=FALSE, "590 nm"=FALSE, "485 nm"=FALSE, "Manual Control"=FALSE} ("Laser Controls 2"), "Initialize"=TRUE) -> ()  [unwired: 11 in, 2 out]
      }
      frame "Start FPGA Acquisition" {
        n531 = Unbundle By Name(w1102) -> ("Scan Mode"=w1101:enum16{"XY", "XZ", "YZ", "XYZ"})
        n532 = case shown="\"XZ\", Default" w1101 {
          tunnel: w1102 -> [_ w1112]
          tunnel: w1100 -> [_ w1113]
          frame "YZ" {
            n533 = vi-ref "FPGA Sample Scanning V1.vi"() -> (w1108:refnum<vi>)
            n534 = property class="VI Interface Type 3"(reference=w1108) -> ("Path"=w1106:path)  [unwired: 1 in, 2 out]
            n535 = Open VI Reference(type specifier VI Refnum (for type only)=w1108, vi path=w1106, options=128) -> (vi reference=w1109:refnum<vi>)  [unwired: 3 in, 1 out]
            n536 = call-by-ref "Start Asynchronous Call"(reference=w1109) -> (reference out=w1110:refnum<vi>)  [unwired: 4 in, 1 out]
            n537 = Close Reference(reference=w1110) -> ()  [unwired: 1 in, 1 out]
          }
          frame "XZ", Default {
            n538 = vi-ref "FPGA Beam Scanning V1.vi"() -> (w1111:refnum<vi>)
            n539 = property class="VI Interface Type 4"(reference=w1111) -> ("Path"=w1115:path)  [unwired: 1 in, 2 out]
            n540 = Open VI Reference(type specifier VI Refnum (for type only)=w1111, vi path=w1115, options=128) -> (vi reference=w1114:refnum<vi>)  [unwired: 3 in, 1 out]
            n541 = call-by-ref "Start Asynchronous Call"(reference=w1114, "Detectors"=w1113, "Image Acquisition Parameters"=w1112) -> (reference out=w1117:refnum<vi>)  [unwired: 2 in, 1 out]
            n542 = Close Reference(reference=w1117) -> ()  [unwired: 1 in, 1 out]
          }
        }
      }
    }
  }
